vi "3 Phase Generator PMU Testing.vi"() -> ()   [LabVIEW 2022 SP3]
uses:
  <vilib>/Utility/TDMS File Viewer/NI_TDMS File Viewer.lvlib
  <vilib>/measure/NI_MAPro.lvlib
  <vilib>/Waveform/WDTOps.llb/WDT Get Waveform Time Array DBL.vi
panel:
  out "Phase 2":picture caption="Phasors visualization"
  in  "Data type":i32=8
  in  "ROCOF":dbl caption="Offset"
  in  "Data save 2":bool
  in  "Data save":bool
  in  "?":enum32{"Test set-up", "Set up"}(tab)
  out "h2rad":string="rad"
  out "h1rad":string="rad"
  out "h2deg\nH2deg":string="deg"
  out "H1deg":string="deg"
  out "H2V":string="V"
  out "H1V":string="V"
  out "H2pu":string="pu"
  out "H1pu":string="pu"
  out "PMrad":string="rad"
  out "PMdeg":string="deg"
  out "PMFeq":string="Hz"
  out "FreqDev":string="Hz"
  out "second":string="s"
  out "Hz/s":string="Hz/s"
  out "Final freq":string="Hz"
  out "Voltage step (V)":string="V"
  out "Voltage step (pu)":string="pu"
  out "?":string="Hz"
  out "AM (V)":string="V"
  out "AM (pu)":string="pu"
  out "?":string="Hz"
  out "?":string="Hz"
  out "?":string="V"
  out "?":string="pu"
  in  "H2 order":dbl=5.0 format="%#_13g"
  in  "Start":bool
  in  "Final freq.":dbl=55.0 format="%.2f"
  in  "ROCOF rate":dbl=1.0 format="%.2f"
  in  "Select test type":u16(ring) items=["Steady state", "Voltage step", "Phase step", "Frequency step", "Frequency ramp", "Amplitude modulation", "Phase modulation", "Harmonics"]
  in  "Frequency step":dbl caption="Offset" min=-5.0 max=5.0 format="%#.6f"
  in  "Phase step":dbl caption="Offset" min=-360.0 max=360.0 format="%#.6f"
  in  "Phase":dbl caption="Offset" min=-360.0 max=360.0
  in  "Voltage":dbl=1.0 caption="Offset" max=1.25 format="%#_5g"
  in  "Voltage step":dbl caption="Offset" min=-0.25 max=0.25 format="%#.6f"
  in  "Frequency":dbl=50.0 caption="Offset" max=55.0 format="%#_7g"
  in  "Mod Freq":dbl=1.0 caption="Offset" min=0.0 max=2.384 step=0.1 format="%#.6f"
  in  "Mod Amp":dbl=0.1 caption="Offset" max=0.125 format="%#.4f"
  in  "Mod Amp":dbl=0.1 caption="Offset" max=15.0 format="%#.4f"
  in  "Mod Freq":dbl=1.0 caption="Offset" format="%#.6f"
  in  "Nominal voltage":dbl=230.0 caption="Offset" format="%_6f"
  in  "stop":bool
  in  "Phase":dbl caption="Offset"
  in  "H1 Volt":dbl=0.05 format="%#_13g"
  in  "H2 Volt":dbl=0.05 format="%#_13g"
  in  "H1 Phase":dbl format="%#_13g"
  in  "H1 order":dbl=3.0 format="%#_13g"
  in  "H2 Phase":dbl format="%#_13g"
  out "Freq Dev":dbl caption="Offset" max=15.0 format="%#.4f"
  out "ROCOF":dbl
  out "Frequency":dbl=50.0 format="%#.8g"
  out "Voltage":dbl=1.0 format="%#_7g"
  out "Phase":dbl
  out "Phase (rad)":string="rad"
  out "Phase (deg)":string="deg"
  out "Time":dbl
  in  "File Name":string="testfile.tdms" caption="File name"
  in  "start":bool
  out "Phase step (rad)":string="rad"
  out "Phase step (deg)":string="deg"
  in  "Nominal Voltage":dbl=230.0 format="%#_13g"
  out "Transmitted Data":string
  in  "Voltage unit":u16(ring)=1 items=["Nominal voltage", "Per-unit voltage"]
  in  "Phase unit":u16(ring) items=["Degree", "Radian"]
  in  "Sampling info":cluster{"Fs":dbl, "#s":dbl}={"Fs"=10000.0, "#s"=1000.0} {"Fs" format="%.2p"}
  in  "LAN Module IP Address":string
  in  "LAN Port":u16
  in  "Nominal Frequency":dbl=50.0 format="%#_13g"
  out "Phase waveform 2":dbl(graph)
  in  "Initial freq.":dbl=50.0 format="%.2f"
  out "ROCOF waveform 2":dbl(graph)
  out "ROCOF waveform":dynamicdata(graph)
  out "Frequency waveform 2":dbl(graph)
  out "Frequency waveform":dynamicdata(graph)
  out "Votlage waveform":dynamicdata(graph)
  out "Numeric":i32
  out "resulting string 2":string
  out "double precision float":dbl[](array[numeric])
  out "Array 3":dbl[](array[numeric])
  out "Array 2":dbl[](array[numeric])
  out "Array":dbl[](array[numeric])
  out "Phase waveform":waveform(dbl)(graph)
  # "Current phasor values"
  # "UDP Protocol"
  # "Waveform scaling"
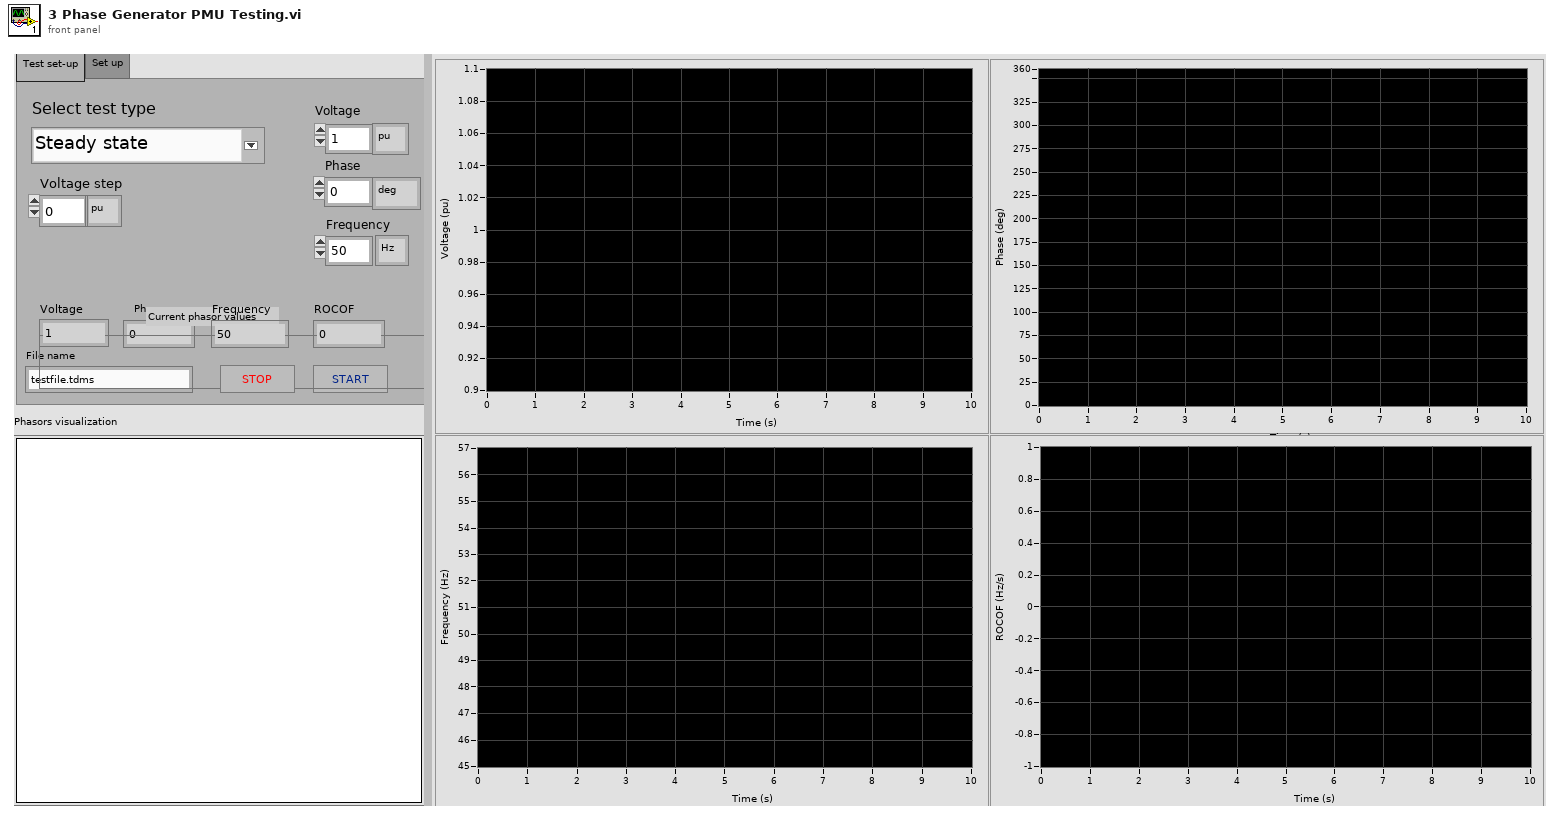
[diagram p1: front panel]
types:
  T1 = enum16{"open", "open or create", "create or replace", "create", "open (read-only)"}
  T2 = cluster{"maximum":dbl, "minimum":dbl, "clip to min":bool, "log?(F)":bool, "grid color":u32, "plot color":u32, "fmt and prec":cluster{"format":enum8{"Decimal", "Scientific", "Engineering", "Binary", "Octal", "Hex"}, "precision":u8}, "visible section":u16}
  T3 = typedef "LVBoundsTypeDef.ctl" = cluster{"Width":u32, "Height":u32}
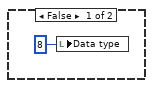
[diagram p2: hidden frame]
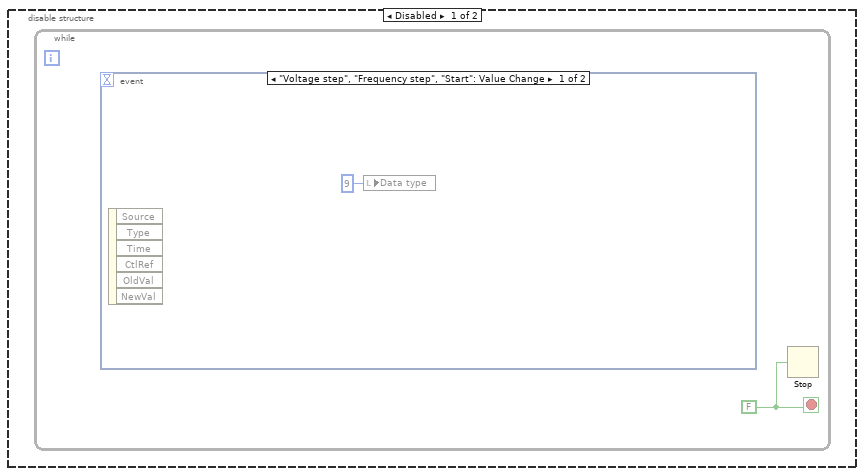
[diagram p3: hidden frame]
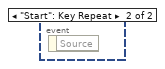
[diagram p4: hidden frame]
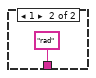
[diagram p5: hidden frame]
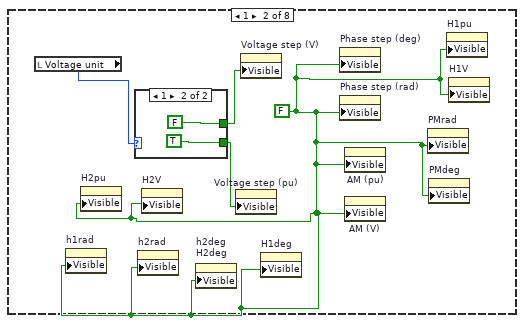
[diagram p6: hidden frame]
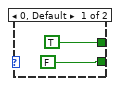
[diagram p7: hidden frame]
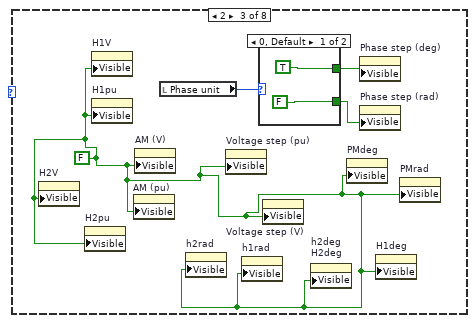
[diagram p8: hidden frame]
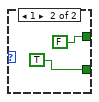
[diagram p9: hidden frame]
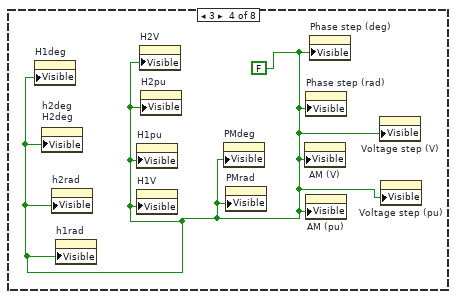
[diagram p10: hidden frame]
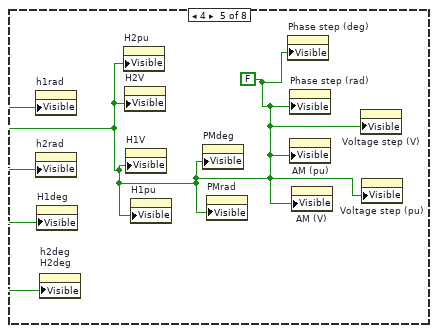
[diagram p11: hidden frame]
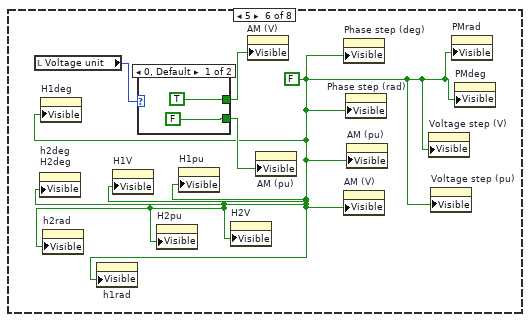
[diagram p12: hidden frame]
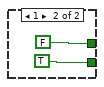
[diagram p13: hidden frame]
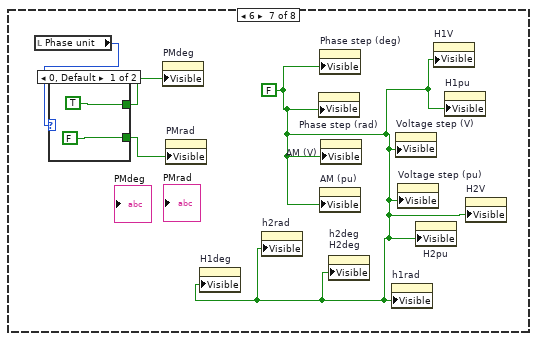
[diagram p14: hidden frame]
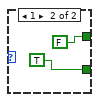
[diagram p15: hidden frame]
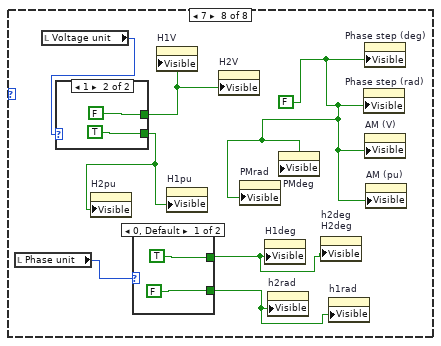
[diagram p16: hidden frame]
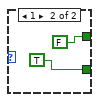
[diagram p17: hidden frame]
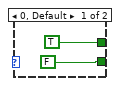
[diagram p18: hidden frame]
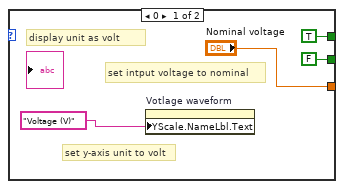
[diagram p19: hidden frame]
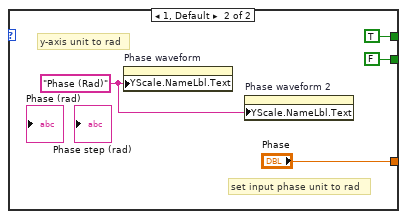
[diagram p20: hidden frame]
diagram:
  n1 = call <vilib>:"Application Directory.vi"() -> ("Application Directory"=w5:path)
  n2 = Concatenate Strings("measurements\\", "File Name") -> (w3:string)
  n3 = Build Path(base path=w5, name or relative path=w3) -> (appended path=w4:path)
  n4 = flat-sequence {
    frame #0 {
      w23 = FALSE
      n5 = local read "Data type"() -> (w29:i32)
      n6 = local read "start"() -> (w22:bool)
      n7 = Equal?(x=w29, y=8) -> (x = y?=w28:bool)
      n8 = Equal?(x=w22, y=TRUE) -> (x = y?=w27:bool)
      n9 = And(x=w27, y=w28) -> (x .and. y?=w26:bool)
      n10 = case shown="True" w26 {
        frame False {
          n11 = local write "Data type"(8 ("Data type")) -> ()
        }
        frame True {
          n12 = local write "Data type"(9 ("Data type")) -> ()
        }
      }
      n13 = property on="Start" class="Bool (strict)"("Value"=w23) -> ()  [unwired: 2 in, 2 out]
      n14 = property on="start" class="Bool (strict)"("Value"=w23) -> ()  [unwired: 2 in, 2 out]
    }
  }
  n15 = TDMS Open(10:T1."create or replace" ("operation (0:open)"), 11:w4) -> (0:w14:errorcluster, 3:w15:refnum<k34>)  [unwired: 5 in]
  n16 = TDMS Set Properties(5:"Data file for PMU testing", 7:"title", 8:w14, 11:w15) -> (0:w12:errorcluster, 3:w13:refnum<k34>)  [unwired: 2 in, 2 out]
  n17 = Get Date/Time In Seconds() -> (seconds since 1Jan1904=w16:timestamp)
  n18 = TDMS Set Properties(5:w16, 7:"datetime", 8:w12, 11:w13) -> (0:w7:errorcluster, 3:w6:refnum<k34>)  [unwired: 2 in, 2 out]
  n19 = while {
    tunnel: [w37] -> w18
    tunnel: [w36] -> w17
    tunnel: w7 -> [w34]
    tunnel: w6 -> [w35]
    i -> [w69]
    stop <- "stop" stop-if-true
    w44 = "3 Phase Generator" ("group name in (Untitled)")
    # "amplitude modulation\nmod freq unit"
    # "phase \nmodulation\namplitude \nunit"
    # "stop button"
    # "box for config layout"
    n20 = flat-sequence {
      tunnel: ["start"] -> w40
      tunnel: ["start"] -> _
      tunnel: [w87] -> w43
      tunnel: [w82] -> w42
      tunnel: [w85] -> w41
      tunnel: w40 -> [w87]
      tunnel: [w166] -> w74
      tunnel: w43 -> [w166]
      tunnel: w42 -> [w160]
      tunnel: w41 -> [w178]
      tunnel: w39 -> [w174]
      tunnel: w38 -> [w173]
      tunnel: [w172] -> w37
      tunnel: [w171] -> w36
      tunnel: w74 -> [w738]
      frame #0 {
        # "input freq unit"
        # "start button"
      }
      frame #1 {
        # "voltage step"
        # "amplitude modulation unit"
        # "set default angle unit ot rad\nif input deg, convert to rad"
        # "enable nominal voltage"
        # "enable unit volt"
        # "enable unit per-unit"
        # "enable per-unit voltage"
        # "per-unit voltage or nominal voltage"
        n21 = local read "Select test type"() -> (w80:u16)
        n22 = case shown="0" "Phase unit" {
          tunnel: [w147 "Phase"] -> w82
          tunnel: [FALSE TRUE] -> w78
          tunnel: [TRUE FALSE] -> w79
          frame 0 {
            # "convert deg to rad"
            # "y-axis in deg"
            # "set input phase unit to deg"
            n23 = property on="Phase waveform" class="WFChart (strict)"("YScale.NameLbl.Text"="Phase (deg)" ("Y Scale.Name Label.Text")) -> ()  [unwired: 2 in, 2 out]
            n24 = Multiply(x="Phase", y=3.141592653589793) -> (x*y=w150:dbl)
            n25 = Divide(x=w150, y=180.0) -> (x/y=w147:dbl)
          }
          frame 1, Default {
            w154 = "Phase (Rad)" ("Y Scale.Name Label.Text")
            # "y-axis unit to rad"
            # "set input phase unit to rad"
            n26 = property on="Phase waveform" class="WFChart (strict)"("YScale.NameLbl.Text"=w154) -> ()  [unwired: 2 in, 2 out]
            n27 = property on="Phase waveform 2" class="WFChart (strict)"("YScale.NameLbl.Text"=w154) -> ()  [unwired: 2 in, 2 out]
          }
        }
        n28 = case shown="0, Default" w80 {
          frame 0, Default {
            w88 = FALSE
            n29 = property on="H2V" class="Str"("Visible"=w88) -> ()  [unwired: 2 in, 2 out]
            n30 = property on="H2pu" class="Str"("Visible"=w88) -> ()  [unwired: 2 in, 2 out]
            n31 = property on="h1rad" class="Str"("Visible"=w88) -> ()  [unwired: 2 in, 2 out]
            n32 = property on="H1deg" class="Str"("Visible"=w88) -> ()  [unwired: 2 in, 2 out]
            n33 = property on="H1V" class="Str"("Visible"=w88) -> ()  [unwired: 2 in, 2 out]
            n34 = property on="H1pu" class="Str"("Visible"=w88) -> ()  [unwired: 2 in, 2 out]
            n35 = property on="h2rad" class="Str"("Visible"=w88) -> ()  [unwired: 2 in, 2 out]
            n36 = property on="h2deg\nH2deg" class="Str"("Visible"=w88) -> ()  [unwired: 2 in, 2 out]
            n37 = property on="PMdeg" class="Str"("Visible"=w88) -> ()  [unwired: 2 in, 2 out]
            n38 = property on="PMrad" class="Str"("Visible"=w88) -> ()  [unwired: 2 in, 2 out]
            n39 = property on="Voltage step (pu)" class="Str"("Visible"=w88) -> ()  [unwired: 2 in, 2 out]
            n40 = property on="AM (pu)" class="Str"("Visible"=w88) -> ()  [unwired: 2 in, 2 out]
            n41 = property on="AM (V)" class="Str"("Visible"=w88) -> ()  [unwired: 2 in, 2 out]
            n42 = property on="Phase step (deg)" class="Str"("Visible"=w88) -> ()  [unwired: 2 in, 2 out]
            n43 = property on="Phase step (rad)" class="Str"("Visible"=w88) -> ()  [unwired: 2 in, 2 out]
            n44 = property on="Voltage step (V)" class="Str"("Visible"=w88) -> ()  [unwired: 2 in, 2 out]
          }
          frame 1 {
            w89 = FALSE
            n45 = local read "Voltage unit"() -> (w92:u16)
            n46 = property on="h1rad" class="Str"("Visible"=w89) -> ()  [unwired: 2 in, 2 out]
            n47 = property on="H2pu" class="Str"("Visible"=w89) -> ()  [unwired: 2 in, 2 out]
            n48 = case shown="1" w92 {
              tunnel: [TRUE FALSE] -> w90
              tunnel: [FALSE TRUE] -> w91
              frame 0, Default {
              }
              frame 1 {
              }
            }
            n49 = property on="h2rad" class="Str"("Visible"=w89) -> ()  [unwired: 2 in, 2 out]
            n50 = property on="H2V" class="Str"("Visible"=w89) -> ()  [unwired: 2 in, 2 out]
            n51 = property on="h2deg\nH2deg" class="Str"("Visible"=w89) -> ()  [unwired: 2 in, 2 out]
            n52 = property on="Voltage step (pu)" class="Str"("Visible"=w91) -> ()  [unwired: 2 in, 2 out]
            n53 = property on="Voltage step (V)" class="Str"("Visible"=w90) -> ()  [unwired: 2 in, 2 out]
            n54 = property on="H1deg" class="Str"("Visible"=w89) -> ()  [unwired: 2 in, 2 out]
            n55 = property on="Phase step (deg)" class="Str"("Visible"=w89) -> ()  [unwired: 2 in, 2 out]
            n56 = property on="Phase step (rad)" class="Str"("Visible"=w89) -> ()  [unwired: 2 in, 2 out]
            n57 = property on="AM (pu)" class="Str"("Visible"=w89) -> ()  [unwired: 2 in, 2 out]
            n58 = property on="AM (V)" class="Str"("Visible"=w89) -> ()  [unwired: 2 in, 2 out]
            n59 = property on="PMrad" class="Str"("Visible"=w89) -> ()  [unwired: 2 in, 2 out]
            n60 = property on="PMdeg" class="Str"("Visible"=w89) -> ()  [unwired: 2 in, 2 out]
            n61 = property on="H1pu" class="Str"("Visible"=w89) -> ()  [unwired: 2 in, 2 out]
            n62 = property on="H1V" class="Str"("Visible"=w89) -> ()  [unwired: 2 in, 2 out]
          }
          frame 2 {
            w97 = FALSE
            n63 = property on="H2V" class="Str"("Visible"=w97) -> ()  [unwired: 2 in, 2 out]
            n64 = property on="H2pu" class="Str"("Visible"=w97) -> ()  [unwired: 2 in, 2 out]
            n65 = property on="H1V" class="Str"("Visible"=w97) -> ()  [unwired: 2 in, 2 out]
            n66 = property on="H1pu" class="Str"("Visible"=w97) -> ()  [unwired: 2 in, 2 out]
            n67 = property on="AM (pu)" class="Str"("Visible"=w97) -> ()  [unwired: 2 in, 2 out]
            n68 = property on="AM (V)" class="Str"("Visible"=w97) -> ()  [unwired: 2 in, 2 out]
            n69 = local read "Phase unit"() -> (w98:u16)
            n70 = property on="h2rad" class="Str"("Visible"=w97) -> ()  [unwired: 2 in, 2 out]
            n71 = property on="Voltage step (pu)" class="Str"("Visible"=w97) -> ()  [unwired: 2 in, 2 out]
            n72 = property on="h1rad" class="Str"("Visible"=w97) -> ()  [unwired: 2 in, 2 out]
            n73 = case shown="0, Default" w98 {
              tunnel: [TRUE FALSE] -> w100
              tunnel: [FALSE TRUE] -> w99
              frame 0, Default {
              }
              frame 1 {
              }
            }
            n74 = property on="Voltage step (V)" class="Str"("Visible"=w97) -> ()  [unwired: 2 in, 2 out]
            n75 = property on="h2deg\nH2deg" class="Str"("Visible"=w97) -> ()  [unwired: 2 in, 2 out]
            n76 = property on="PMdeg" class="Str"("Visible"=w97) -> ()  [unwired: 2 in, 2 out]
            n77 = property on="Phase step (deg)" class="Str"("Visible"=w100) -> ()  [unwired: 2 in, 2 out]
            n78 = property on="Phase step (rad)" class="Str"("Visible"=w99) -> ()  [unwired: 2 in, 2 out]
            n79 = property on="H1deg" class="Str"("Visible"=w97) -> ()  [unwired: 2 in, 2 out]
            n80 = property on="PMrad" class="Str"("Visible"=w97) -> ()  [unwired: 2 in, 2 out]
          }
          frame 3 {
            w105 = FALSE
            n81 = property on="H1deg" class="Str"("Visible"=w105) -> ()  [unwired: 2 in, 2 out]
            n82 = property on="h2deg\nH2deg" class="Str"("Visible"=w105) -> ()  [unwired: 2 in, 2 out]
            n83 = property on="h2rad" class="Str"("Visible"=w105) -> ()  [unwired: 2 in, 2 out]
            n84 = property on="h1rad" class="Str"("Visible"=w105) -> ()  [unwired: 2 in, 2 out]
            n85 = property on="H1pu" class="Str"("Visible"=w105) -> ()  [unwired: 2 in, 2 out]
            n86 = property on="H1V" class="Str"("Visible"=w105) -> ()  [unwired: 2 in, 2 out]
            n87 = property on="H2V" class="Str"("Visible"=w105) -> ()  [unwired: 2 in, 2 out]
            n88 = property on="H2pu" class="Str"("Visible"=w105) -> ()  [unwired: 2 in, 2 out]
            n89 = property on="PMdeg" class="Str"("Visible"=w105) -> ()  [unwired: 2 in, 2 out]
            n90 = property on="PMrad" class="Str"("Visible"=w105) -> ()  [unwired: 2 in, 2 out]
            n91 = property on="AM (V)" class="Str"("Visible"=w105) -> ()  [unwired: 2 in, 2 out]
            n92 = property on="Phase step (rad)" class="Str"("Visible"=w105) -> ()  [unwired: 2 in, 2 out]
            n93 = property on="AM (pu)" class="Str"("Visible"=w105) -> ()  [unwired: 2 in, 2 out]
            n94 = property on="Phase step (deg)" class="Str"("Visible"=w105) -> ()  [unwired: 2 in, 2 out]
            n95 = property on="Voltage step (V)" class="Str"("Visible"=w105) -> ()  [unwired: 2 in, 2 out]
            n96 = property on="Voltage step (pu)" class="Str"("Visible"=w105) -> ()  [unwired: 2 in, 2 out]
          }
          frame 4 {
            w106 = FALSE
            n97 = property on="h1rad" class="Str"("Visible"=w106) -> ()  [unwired: 2 in, 2 out]
            n98 = property on="h2rad" class="Str"("Visible"=w106) -> ()  [unwired: 2 in, 2 out]
            n99 = property on="H1deg" class="Str"("Visible"=w106) -> ()  [unwired: 2 in, 2 out]
            n100 = property on="h2deg\nH2deg" class="Str"("Visible"=w106) -> ()  [unwired: 2 in, 2 out]
            n101 = property on="H2pu" class="Str"("Visible"=w106) -> ()  [unwired: 2 in, 2 out]
            n102 = property on="H2V" class="Str"("Visible"=w106) -> ()  [unwired: 2 in, 2 out]
            n103 = property on="H1V" class="Str"("Visible"=w106) -> ()  [unwired: 2 in, 2 out]
            n104 = property on="H1pu" class="Str"("Visible"=w106) -> ()  [unwired: 2 in, 2 out]
            n105 = property on="PMdeg" class="Str"("Visible"=w106) -> ()  [unwired: 2 in, 2 out]
            n106 = property on="PMrad" class="Str"("Visible"=w106) -> ()  [unwired: 2 in, 2 out]
            n107 = property on="Phase step (deg)" class="Str"("Visible"=w106) -> ()  [unwired: 2 in, 2 out]
            n108 = property on="Phase step (rad)" class="Str"("Visible"=w106) -> ()  [unwired: 2 in, 2 out]
            n109 = property on="AM (pu)" class="Str"("Visible"=w106) -> ()  [unwired: 2 in, 2 out]
            n110 = property on="AM (V)" class="Str"("Visible"=w106) -> ()  [unwired: 2 in, 2 out]
            n111 = property on="Voltage step (V)" class="Str"("Visible"=w106) -> ()  [unwired: 2 in, 2 out]
            n112 = property on="Voltage step (pu)" class="Str"("Visible"=w106) -> ()  [unwired: 2 in, 2 out]
          }
          frame 5 {
            w107 = FALSE
            n113 = local read "Voltage unit"() -> (w110:u16)
            n114 = property on="h2deg\nH2deg" class="Str"("Visible"=w107) -> ()  [unwired: 2 in, 2 out]
            n115 = property on="H1deg" class="Str"("Visible"=w107) -> ()  [unwired: 2 in, 2 out]
            n116 = property on="h2rad" class="Str"("Visible"=w107) -> ()  [unwired: 2 in, 2 out]
            n117 = property on="h1rad" class="Str"("Visible"=w107) -> ()  [unwired: 2 in, 2 out]
            n118 = property on="H1V" class="Str"("Visible"=w107) -> ()  [unwired: 2 in, 2 out]
            n119 = case shown="0, Default" w110 {
              tunnel: [TRUE FALSE] -> w109
              tunnel: [FALSE TRUE] -> w108
              frame 0, Default {
              }
              frame 1 {
              }
            }
            n120 = property on="H2pu" class="Str"("Visible"=w107) -> ()  [unwired: 2 in, 2 out]
            n121 = property on="H1pu" class="Str"("Visible"=w107) -> ()  [unwired: 2 in, 2 out]
            n122 = property on="H2V" class="Str"("Visible"=w107) -> ()  [unwired: 2 in, 2 out]
            n123 = property on="AM (V)" class="Str"("Visible"=w109) -> ()  [unwired: 2 in, 2 out]
            n124 = property on="AM (pu)" class="Str"("Visible"=w108) -> ()  [unwired: 2 in, 2 out]
            n125 = property on="Phase step (deg)" class="Str"("Visible"=w107) -> ()  [unwired: 2 in, 2 out]
            n126 = property on="AM (V)" class="Str"("Visible"=w107) -> ()  [unwired: 2 in, 2 out]
            n127 = property on="Phase step (rad)" class="Str"("Visible"=w107) -> ()  [unwired: 2 in, 2 out]
            n128 = property on="AM (pu)" class="Str"("Visible"=w107) -> ()  [unwired: 2 in, 2 out]
            n129 = property on="Voltage step (V)" class="Str"("Visible"=w107) -> ()  [unwired: 2 in, 2 out]
            n130 = property on="Voltage step (pu)" class="Str"("Visible"=w107) -> ()  [unwired: 2 in, 2 out]
            n131 = property on="PMrad" class="Str"("Visible"=w107) -> ()  [unwired: 2 in, 2 out]
            n132 = property on="PMdeg" class="Str"("Visible"=w107) -> ()  [unwired: 2 in, 2 out]
          }
          frame 6 {
            w115 = FALSE
            n133 = local read "Phase unit"() -> (w118:u16)
            n134 = case shown="0, Default" w118 {
              tunnel: [TRUE FALSE] -> w117
              tunnel: [FALSE TRUE] -> w116
              frame 0, Default {
              }
              frame 1 {
              }
            }
            n135 = property on="PMdeg" class="Str"("Visible"=w117) -> ()  [unwired: 2 in, 2 out]
            n136 = property on="PMrad" class="Str"("Visible"=w116) -> ()  [unwired: 2 in, 2 out]
            n137 = property on="H1deg" class="Str"("Visible"=w115) -> ()  [unwired: 2 in, 2 out]
            n138 = property on="h2rad" class="Str"("Visible"=w115) -> ()  [unwired: 2 in, 2 out]
            n139 = property on="Phase step (rad)" class="Str"("Visible"=w115) -> ()  [unwired: 2 in, 2 out]
            n140 = property on="Phase step (deg)" class="Str"("Visible"=w115) -> ()  [unwired: 2 in, 2 out]
            n141 = property on="AM (pu)" class="Str"("Visible"=w115) -> ()  [unwired: 2 in, 2 out]
            n142 = property on="AM (V)" class="Str"("Visible"=w115) -> ()  [unwired: 2 in, 2 out]
            n143 = property on="h2deg\nH2deg" class="Str"("Visible"=w115) -> ()  [unwired: 2 in, 2 out]
            n144 = property on="h1rad" class="Str"("Visible"=w115) -> ()  [unwired: 2 in, 2 out]
            n145 = property on="Voltage step (V)" class="Str"("Visible"=w115) -> ()  [unwired: 2 in, 2 out]
            n146 = property on="Voltage step (pu)" class="Str"("Visible"=w115) -> ()  [unwired: 2 in, 2 out]
            n147 = property on="H2pu" class="Str"("Visible"=w115) -> ()  [unwired: 2 in, 2 out]
            n148 = property on="H1V" class="Str"("Visible"=w115) -> ()  [unwired: 2 in, 2 out]
            n149 = property on="H1pu" class="Str"("Visible"=w115) -> ()  [unwired: 2 in, 2 out]
            n150 = property on="H2V" class="Str"("Visible"=w115) -> ()  [unwired: 2 in, 2 out]
          }
          frame 7 {
            w129 = FALSE
            n151 = local read "Phase unit"() -> (w123:u16)
            n152 = local read "Voltage unit"() -> (w128:u16)
            n153 = case shown="1" w128 {
              tunnel: [TRUE FALSE] -> w127
              tunnel: [FALSE TRUE] -> w126
              frame 0, Default {
              }
              frame 1 {
              }
            }
            n154 = property on="H2pu" class="Str"("Visible"=w126) -> ()  [unwired: 2 in, 2 out]
            n155 = case shown="0, Default" w123 {
              tunnel: [TRUE FALSE] -> w125
              tunnel: [FALSE TRUE] -> w124
              frame 0, Default {
              }
              frame 1 {
              }
            }
            n156 = property on="H1V" class="Str"("Visible"=w127) -> ()  [unwired: 2 in, 2 out]
            n157 = property on="H1pu" class="Str"("Visible"=w126) -> ()  [unwired: 2 in, 2 out]
            n158 = property on="H2V" class="Str"("Visible"=w127) -> ()  [unwired: 2 in, 2 out]
            n159 = property on="PMrad" class="Str"("Visible"=w129) -> ()  [unwired: 2 in, 2 out]
            n160 = property on="H1deg" class="Str"("Visible"=w125) -> ()  [unwired: 2 in, 2 out]
            n161 = property on="h2rad" class="Str"("Visible"=w124) -> ()  [unwired: 2 in, 2 out]
            n162 = property on="PMdeg" class="Str"("Visible"=w129) -> ()  [unwired: 2 in, 2 out]
            n163 = property on="h2deg\nH2deg" class="Str"("Visible"=w125) -> ()  [unwired: 2 in, 2 out]
            n164 = property on="h1rad" class="Str"("Visible"=w124) -> ()  [unwired: 2 in, 2 out]
            n165 = property on="Phase step (rad)" class="Str"("Visible"=w129) -> ()  [unwired: 2 in, 2 out]
            n166 = property on="Phase step (deg)" class="Str"("Visible"=w129) -> ()  [unwired: 2 in, 2 out]
            n167 = property on="AM (V)" class="Str"("Visible"=w129) -> ()  [unwired: 2 in, 2 out]
            n168 = property on="AM (pu)" class="Str"("Visible"=w129) -> ()  [unwired: 2 in, 2 out]
          }
        }
        n169 = case shown="1, Default" "Voltage unit" {
          tunnel: ["Nominal voltage" "Voltage"] -> w85
          tunnel: [TRUE FALSE] -> w83
          tunnel: [FALSE TRUE] -> w84
          frame 0 {
            # "set intput voltage to nominal"
            # "display unit as volt"
            # "set y-axis unit to volt"
            n170 = property on="Votlage waveform" class="WFChart (strict)"("YScale.NameLbl.Text"="Voltage (V)" ("Y Scale.Name Label.Text")) -> ()  [unwired: 2 in, 2 out]
          }
          frame 1, Default {
            # "set voltage unit to pu"
            # "set y-axis to show in per-unit scale"
            n171 = property on="Votlage waveform" class="WFChart (strict)"("YScale.NameLbl.Text"="Voltage (pu)" ("Y Scale.Name Label.Text")) -> ()  [unwired: 2 in, 2 out]
          }
        }
        n172 = property on="AM (pu)" class="Str" props=["Visible"]() -> ()  [unwired: 2 in, 3 out]
        n173 = property on="AM (pu)" class="Str" props=["Visible"]() -> ()  [unwired: 2 in, 3 out]
        n174 = property on="Phase (deg)" class="Str"("Visible"=w79) -> ()  [unwired: 2 in, 2 out]
        n175 = property on="Phase (rad)" class="Str"("Visible"=w78) -> ()  [unwired: 2 in, 2 out]
        n176 = property class="Str"("Visible"=w84) -> ()  [unwired: 2 in, 2 out]
        n177 = property on="Nominal voltage" class="DigNum (strict)"("Visible"=w83) -> ()  [unwired: 2 in, 2 out]
        n178 = property class="Str"("Visible"=w83) -> ()  [unwired: 2 in, 2 out]
        n179 = property on="Voltage" class="DigNum (strict)"("Visible"=w84) -> ()  [unwired: 2 in, 2 out]
        n180 = property on="Phase (rad)" class="DigNum (strict)"("Visible"=w78) -> ()  [unwired: 2 in, 2 out]
        n181 = property on="Phase (deg)" class="DigNum (strict)"("Visible"=w79) -> ()  [unwired: 2 in, 2 out]
        n182 = invoke on="double precision float" class="Arr (strict)" method="Reinit To Default"() -> ()  [unwired: 3 in, 3 out]
      }
      frame #2 {
        # "phase in"
        # "voltage in"
        # "start generating"
        n183 = invoke on="Array 3" class="Arr (strict)" method="Reinit To Default"() -> ()  [unwired: 3 in, 3 out]
        n184 = invoke on="Array 2" class="Arr (strict)" method="Reinit To Default"() -> ()  [unwired: 3 in, 3 out]
        n185 = invoke on="Array" class="Arr (strict)" method="Reinit To Default"() -> ()  [unwired: 3 in, 3 out]
        n186 = case shown="True" w166 {
          selector: w166 -> [_ w255]
          tunnel: "Select test type" -> [w224 w263]
          tunnel: [w220 w260] -> w163
          tunnel: [w223 w251] -> w176
          tunnel: [w218 w248] -> _
          tunnel: [w217 w252] -> w158
          tunnel: [w215 w249] -> w164
          tunnel: [w219 w250] -> w165
          tunnel: [w216 w259] -> w159
          tunnel: [w221 w258] -> _
          tunnel: [w222 w257] -> w162
          tunnel: [w209 w256] -> w161
          tunnel: w160 -> [_ w254]
          tunnel: w178 -> [_ w253]
          tunnel: [w214 w247] -> w177
          tunnel: [w213 w246] -> w175
          tunnel: [w212 w245] -> w170
          tunnel: [w212 w244] -> w169
          tunnel: [w212 w243] -> w168
          tunnel: [w212 w242] -> w167
          frame False {
            w210 = dbl[] [] ("History Data")
            w212 = dbl[] []
            w211 = waveform(dbl)[] [] ("History Data")
            n187 = property on="Frequency waveform 2" class="WFChart (strict)"("History Data"=w210) -> ()  [unwired: 2 in, 2 out]
            n188 = property on="ROCOF waveform 2" class="WFChart (strict)"("History Data"=w210) -> ()  [unwired: 2 in, 2 out]
            n189 = property on="Phase waveform 2" class="WFChart (strict)"("History Data"=w210) -> ()  [unwired: 2 in, 2 out]
            n190 = property on="Frequency waveform" class="WFChart (strict)"("History Data"=w211) -> ()  [unwired: 2 in, 2 out]
            n191 = property on="Phase waveform" class="WFChart (strict)"("History Data"=w211) -> ()  [unwired: 2 in, 2 out]
            n192 = property on="Votlage waveform" class="WFChart (strict)"("History Data"=w211) -> ()  [unwired: 2 in, 2 out]
            n193 = property on="ROCOF waveform" class="WFChart (strict)"("History Data"=w211) -> ()  [unwired: 2 in, 2 out]
            n194 = case shown="0, Default" w224 {
              tunnel: [w226 w228 w229 w231 w234 w236 w238 w239] -> _
              tunnel: [w226 w228 w229 w231 w234 w236 w238 w240] -> w223
              tunnel: [w225 w227 w230 w232 w233 w236 w237 w239] -> w222
              tunnel: [w225 w227 w230 w232 w233 w235 w238 w239] -> w209
              tunnel: [w225 w227 w230 w232 w233 w235 w237 w239] -> w221
              tunnel: [w225 w227 w229 w232 w233 w235 w237 w239] -> w220
              tunnel: [w225 w227 w230 w231 w233 w235 w237 w239] -> w219
              tunnel: [w225 w227 w230 w232 w233 w235 w237 w239] -> w218
              tunnel: [w225 w227 w230 w232 w233 w235 w237 w240] -> w215
              tunnel: [w225 w228 w230 w232 w233 w235 w237 w239] -> w217
              tunnel: [w225 w227 w230 w232 w234 w235 w237 w239] -> w216
              tunnel: [w225 w227 w229 w232 w233 w235 w237 w239] -> w214
              tunnel: [w225 w227 w229 w231 w233 w235 w237 w239] -> w213
              frame 0, Default {
                w226 = TRUE
                w225 = FALSE
              }
              frame 1 {
                w228 = TRUE
                w227 = FALSE
              }
              frame 2 {
                w229 = TRUE
                w230 = FALSE
              }
              frame 3 {
                w231 = TRUE
                w232 = FALSE
              }
              frame 4 {
                w234 = TRUE
                w233 = FALSE
              }
              frame 5 {
                w236 = TRUE
                w235 = FALSE
              }
              frame 6 {
                w238 = TRUE
                w237 = FALSE
              }
              frame 7 {
                w239 = FALSE
                w240 = TRUE
              }
            }
          }
          frame True {
            # "phase mod freq dev unit"
            # "phase mod freq unit"
            n195 = case shown="0, Default" w263 {
              tunnel: w253 -> [w296 w319 w380 w447 w550 w636 w707 w735]
              tunnel: w254 -> [w274 w304 w378 w456 w563 w651 w682 _]
              tunnel: "Frequency" -> [w275 w306 w362 w461 w545 w648 w683 w737]
              tunnel: "ROCOF" -> [w290 w323 w358 w440 _ w647 w681 _]
              tunnel: [w279 w333 w369 w446 w579 w659 w713 w734] -> _
              tunnel: [w289 w311 w369 w449 w546 w634 w680 w734] -> w260
              tunnel: [w279 w333 w369 w446 w579 w659 w713 w736] -> w251
              tunnel: [w289 w311 w369 w449 w546 w659 w713 w736] -> w248
              tunnel: [w279 w333 w369 w446 w579 w659 w713 w734] -> _
              tunnel: [w289 w311 w392 w449 w546 w634 w680 w736] -> w249
              tunnel: [w289 w311 w392 w446 w546 w634 w680 w734] -> w250
              tunnel: [w289 w311 w392 w449 w579 w634 w680 w734] -> w259
              tunnel: [w289 w311 w392 w449 w546 w634 w680 w734] -> w258
              tunnel: [w289 w311 w392 w449 w546 w659 w680 w734] -> w257
              tunnel: [w289 w311 w392 w449 w546 w634 w713 w734] -> w256
              tunnel: w255 -> [_ _ _ _ _ _ _ _]
              tunnel: [w289 w333 w392 w449 w546 w634 w680 w734] -> w252
              tunnel: [w289 w311 w369 w449 w546 w634 w680 w734] -> w247
              tunnel: [w279 w311 w369 w446 w546 w634 w680 w734] -> w246
              tunnel: [w285 w307 w365 w435 w539 w630 w676 w733] -> w245
              tunnel: [w286 w309 w363 w444 w544 w629 w673 w733] -> w244
              tunnel: [w266 w308 w364 w436 w542 w632 w674 w733] -> w243
              tunnel: [w277 w310 w366 w443 w528 w631 w675 w733] -> w242
              tunnel: "Nominal Frequency" -> [w267 w305 w339 _ _ _ _ _]
              frame 0, Default {
                w279 = TRUE
                w289 = FALSE
                # "nominal freq"
                # "delta rocof = differenciate delta freq"
                # "rocof func: f(t)=rocof"
                # "input freq: f(t)=f_in"
                # "voltage in func: f(t)=v_in"
                # "Steady state"
                n196 = local read "Sampling info"() -> (w264:cluster{"Fs":dbl, "#s":dbl})
                n197 = local read "Phase unit"() -> (w273:u16)
                n198 = call "phasePlotWrap.vi"("Sampling info"=w264, "Phase unit"=w273, "Phase"=w274, "Nominal Frequency"=w267, "Frequency"=w275) -> ("yScaleMin"=w270:dbl, "yScaleMax"=w271:dbl, "Phase waveform"=w272:waveform(dbl))  [unwired: 4 in]
                "Phase waveform" <- w272
                n199 = call "Convert to Dynamic Data"("Array"=w272) -> ("Dynamic Data Type"=w276:dynamicdata)  [unwired: 3 in]
                n200 = call "Convert from Dynamic Data13"("Dynamic Data Type"=w276) -> ("Array"=w285:dbl[])  [unwired: 3 in]
                n201 = call <vilib>:"Formula Waveform.vi"("sampling info"=w264, "formula"="a", "amplitude"=w275) -> ("signal out"=w266:waveform(dbl))  [unwired: 7 in, 1 out]
                n202 = call <vilib>:"Formula Waveform.vi"("sampling info"=w264, "formula"="a", "frequency"=w267) -> ("signal out"=w268:waveform(dbl))  [unwired: 7 in, 1 out]
                n203 = Subtract(1:w268, 2:w266) -> (0:w265:waveform(dbl))  [unwired: 1 in, 1 out]
                n204 = property on="Phase waveform" class="WFChart (strict)"("YScale.Maximum"=w271) -> ()  [unwired: 2 in, 2 out]
                n205 = property on="Phase waveform" class="WFChart (strict)"("YScale.Minimum"=w270) -> ()  [unwired: 2 in, 2 out]
                n206 = call "Sample Compression8"("Signals"=w266) -> ("Maximum"=w291:dynamicdata)  [unwired: 8 in, 2 out]
                "Frequency waveform" <- w291
                n207 = call "Derivative (dX/dt)"("Signals"=w265) -> ("Result"=w278:dynamicdata)  [unwired: 5 in, 1 out]
                n208 = call "Convert from Dynamic Data3"("Dynamic Data Type"=w278) -> ("Array"=w277:dbl[])  [unwired: 3 in]
                n209 = call <vilib>:"Formula Waveform.vi"("sampling info"=w264, "formula"="a", "amplitude"=w290) -> ("signal out"=w288:waveform(dbl))  [unwired: 7 in, 1 out]
                n210 = local write "Phase"(w272) -> ()
                n211 = call-poly <vilib>:"Get Waveform Time Array.vi"("waveform in"=w288) -> ("X array"=w293:timestamp[])  [unwired: 9 in, 1 out]
                n212 = local write "Frequency"(w291) -> ()
                n213 = call <vilib>:"Formula Waveform.vi"("sampling info"=w264, "formula"="a", "amplitude"=w296) -> ("signal out"=w286:waveform(dbl))  [unwired: 7 in, 1 out]
                n214 = To Double Precision Float(number=w293) -> (double precision float=→"double precision float":dbl[])
                n215 = call "Sample Compression6"("Signals"=w286) -> ("Maximum"=w292:dynamicdata)  [unwired: 8 in, 2 out]
                "Votlage waveform" <- w292
                n216 = call "Sample Compression50"("Signals"=w278) -> ("Maximum"=w280:dynamicdata)  [unwired: 8 in, 2 out]
                "ROCOF" <- w280
                n217 = call "Convert from Dynamic Data10"("Dynamic Data Type"=w280) -> ("Scalar"=w284:dbl)  [unwired: 3 in]
                n218 = local write "Voltage"(w292) -> ()
                n219 = In Range and Coerce(upper limit=5.0, x=w284, lower limit=-5.0) -> (coerced(x)=w281:dbl)  [unwired: 1 out]
                n220 = local write "ROCOF waveform 2"(w281) -> ()
                n221 = call "Elapsed Time3"() -> ("Time has Elapsed"=w287:bool)  [unwired: 12 in, 7 out]
                n222 = Stop(stop? (T)=w287) -> ()
              }
              frame 1 {
                w311 = FALSE
                w333 = TRUE ("Visible")
                # "because the compression remove half of the sample so the last 0.1s will turn to 0.05s, delay 1s will be 0.95s instead"
                # "input freq"
                # "initial phase"
                # "percentage of the base voltage"
                # "base voltage"
                # "voltage step"
                n223 = local read "Sampling info"() -> (w302:cluster{"Fs":dbl, "#s":dbl})
                n224 = call <vilib>:"Formula Waveform.vi"("sampling info"=w302, "formula"="a", "amplitude"=w306) -> ("signal out"=w308:waveform(dbl))  [unwired: 7 in, 1 out]
                n225 = call <vilib>:"Formula Waveform.vi"("sampling info"=w302, "formula"="a", "amplitude"=w304) -> ("signal out"=w307:waveform(dbl))  [unwired: 7 in, 1 out]
                n226 = call "Sample Compression9"("Signals"=w308) -> ("Maximum"=w316:dynamicdata)  [unwired: 8 in, 2 out]
                n227 = local write "Array 2"(w307) -> ()
                n228 = call <vilib>:"Formula Waveform.vi"("sampling info"=w302, "formula"="a", "amplitude"=w319) -> ("signal out"=w313:waveform(dbl))  [unwired: 7 in, 1 out]
                n229 = call <vilib>:"Formula Waveform.vi"("sampling info"=w302, "formula"="a", "amplitude"=w323) -> ("signal out"=w310:waveform(dbl))  [unwired: 7 in, 1 out]
                n230 = call <vilib>:"Formula Waveform.vi"("sampling info"=w302, "formula"="a+a*f", "amplitude"=w319, "frequency"="Voltage step") -> ("signal out"=w315:waveform(dbl))  [unwired: 6 in, 1 out]
                n231 = local write "Frequency waveform"(w316) -> ()
                n232 = local write "Frequency"(w316) -> ()
                n233 = local write "Array 3"(w308) -> ()
                n234 = call "Sample Compression11"("Signals"=w310) -> ("Maximum"=w317:dynamicdata)  [unwired: 8 in, 2 out]
                n235 = call "Sample Compression12"("Signals"=w313) -> ("Maximum"=w312:dynamicdata)  [unwired: 8 in, 2 out]
                n236 = call "Sample Compression4"("Signals"=w315) -> ("Maximum"=w314:dynamicdata)  [unwired: 8 in, 2 out]
                n237 = local write "ROCOF waveform"(w317) -> ()
                n238 = local write "ROCOF"(w317) -> ()
                n239 = local read "Phase unit"() -> (w303:u16)
                n240 = call "Elapsed Time"() -> ("Elapsed Time (s)"=w332:dbl)  [unwired: 12 in, 7 out]
                n241 = call "phasePlotWrap.vi"("Sampling info"=w302, "Phase unit"=w303, "Phase"=w304, "Nominal Frequency"=w305, "Frequency"=w306) -> ("yScaleMin"=w299:dbl, "yScaleMax"=w300:dbl, "Phase waveform"=w301:waveform(dbl))  [unwired: 4 in]
                n242 = Less Or Equal?(x=w332, y=0.95) -> (x <= y?=w330:bool)
                n243 = local write "Phase waveform"(w301) -> ()
                n244 = property on="Phase waveform" class="WFChart (strict)"("YScale.Maximum"=w300) -> ()  [unwired: 2 in, 2 out]
                n245 = property on="Phase waveform" class="WFChart (strict)"("YScale.Minimum"=w299) -> ()  [unwired: 2 in, 2 out]
                n246 = local write "Phase"(w301) -> ()
                n247 = case shown="False" w330 {
                  tunnel: [w335 w337] -> w318
                  tunnel: w312 -> [_ w337]
                  tunnel: w314 -> [w335 _]
                  tunnel: [w334 w336] -> w309
                  tunnel: w313 -> [_ w336]
                  tunnel: w315 -> [w334 _]
                  frame False {
                  }
                  frame True {
                  }
                }
                "Voltage" <- w318
                "Array" <- w309
                n248 = local write "Votlage waveform"(w318) -> ()
                n249 = call-poly <vilib>:"Get Waveform Time Array.vi"("waveform in"=w309) -> ("X array"=w327:timestamp[])  [unwired: 9 in, 1 out]
                n250 = To Double Precision Float(number=w327) -> (double precision float=w328:dbl[])
                n251 = local write "double precision float"(w328) -> ()
                n252 = call "Elapsed Time2"() -> ("Time has Elapsed"=w329:bool)  [unwired: 12 in, 7 out]
                n253 = Stop(stop? (T)=w329) -> ()
              }
              frame 2 {
                w369 = TRUE
                w392 = FALSE ("Visible")
                # "phase step"
                # "nominal frequency"
                # "input voltage"
                # "input frequency"
                # "because the compression remove half of the sample so the last 0.1s will turn to 0.05s, delay 1s will be 0.95s instead"
                # "initial phase"
                n254 = local read "Sampling info"() -> (w340:cluster{"Fs":dbl, "#s":dbl})
                n255 = call <vilib>:"Formula Waveform.vi"("sampling info"=w340, "formula"="a", "amplitude"=w380) -> ("signal out"=w363:waveform(dbl))  [unwired: 7 in, 1 out]
                n256 = call <vilib>:"Formula Waveform.vi"("sampling info"=w340, "formula"="a", "amplitude"=w358) -> ("signal out"=w355:waveform(dbl))  [unwired: 7 in, 1 out]
                n257 = call <vilib>:"Formula Waveform.vi"("sampling info"=w340, "formula"="a", "amplitude"=w339) -> ("signal out"=w338:waveform(dbl))  [unwired: 7 in, 1 out]
                n258 = local write "Array"(w363) -> ()
                n259 = call <vilib>:"Formula Waveform.vi"("sampling info"=w340, "formula"="a", "amplitude"=w362) -> ("signal out"=w344:waveform(dbl))  [unwired: 7 in, 1 out]
                n260 = call-poly <vilib>:"Get Waveform Time Array.vi"("waveform in"=w363) -> ("X array"=w388:timestamp[])  [unwired: 9 in, 1 out]
                n261 = call "Sample Compression14"("Signals"=w363) -> ("Maximum"=w373:dynamicdata)  [unwired: 8 in, 2 out]
                n262 = call <vilib>:"Formula Waveform.vi"("sampling info"=w340, "formula"="a", "amplitude"=w378) -> ("signal out"=w368:waveform(dbl))  [unwired: 7 in, 1 out]
                n263 = call <vilib>:"Formula Waveform.vi"("sampling info"=w340, "formula"="a+1*f", "amplitude"=w378, "frequency"="Phase step") -> ("signal out"=w375:waveform(dbl))  [unwired: 6 in, 1 out]
                n264 = To Double Precision Float(number=w388) -> (double precision float=w387:dbl[])
                n265 = call "Sample Compression18"("Signals"=w355) -> ("Maximum"=w356:dynamicdata)  [unwired: 8 in, 2 out]
                n266 = call "Sample Compression17"("Signals"=w344) -> ("Maximum"=w360:dynamicdata)  [unwired: 8 in, 2 out]
                n267 = call "Sample Compression48"("Signals"=w338) -> ()  [unwired: 8 in, 3 out]
                n268 = call "Sample Compression15"("Signals"=w375) -> ("Maximum"=w374:dynamicdata)  [unwired: 8 in, 2 out]
                n269 = local write "double precision float"(w387) -> ()
                n270 = call "Sample Compression41"("Signals"=w368) -> ("Maximum"=w376:dynamicdata)  [unwired: 8 in, 2 out]
                n271 = local write "Voltage"(w373) -> ()
                n272 = local write "Votlage waveform"(w373) -> ()
                n273 = call "Elapsed Time4"() -> ("Elapsed Time (s)"=w393:dbl)  [unwired: 12 in, 7 out]
                n274 = Less Or Equal?(x=w393, y=0.95) -> (x <= y?=w357:bool)
                n275 = case shown="False" w357 {
                  tunnel: [w405 w407] -> w347
                  tunnel: w376 -> [_ w407]
                  tunnel: w374 -> [w405 _]
                  tunnel: w368 -> [_ w406]
                  tunnel: [w404 w406] -> w365
                  tunnel: w375 -> [w404 _]
                  frame False {
                  }
                  frame True {
                  }
                }
                "Array 2" <- w365
                n276 = Subtract(1:w368, 2:w365) -> (0:w367:waveform(dbl))  [unwired: 1 in, 1 out]
                n277 = call "Derivative (dX/dt)"("Signals"=w367) -> ("Result"=w345:dynamicdata)  [unwired: 5 in, 1 out]
                n278 = local read "Phase unit"() -> (w346:u16)
                n279 = Add(1:w344, 2:w345) -> (0:w343:dynamicdata)  [unwired: 1 in, 1 out]
                n280 = case shown="0, Default" w346 {
                  tunnel: w347 -> [w394 w395]
                  tunnel: [w394 w395] -> w342
                  frame 0, Default {
                  }
                  frame 1 {
                  }
                }
                "Phase" <- w342
                n281 = call "Sample Compression13"("Signals"=w343) -> ("Maximum"=w349:dynamicdata)  [unwired: 6 in, 4 out]
                n282 = case shown="False" w357 {
                  tunnel: w344 -> [_ w403]
                  tunnel: w360 -> [_ w402]
                  tunnel: [w401 w403] -> w351
                  tunnel: [w400 w402] -> w350
                  tunnel: w343 -> [w401 _]
                  tunnel: w349 -> [w400 _]
                  frame False {
                  }
                  frame True {
                  }
                }
                n283 = call "Convert from Dynamic Data7"("Dynamic Data Type"=w351) -> ("Array"=w364:dbl[])  [unwired: 3 in]
                n284 = local write "Phase waveform"(w342) -> ()
                n285 = call "Derivative (dX/dt)"("Signals"=w351) -> ("Result"=w353:dynamicdata)  [unwired: 5 in, 1 out]
                n286 = call "Elapsed Time5"() -> ("Time has Elapsed"=w391:bool)  [unwired: 12 in, 7 out]
                n287 = call "Convert from Dynamic Data"("Dynamic Data Type"=w350) -> ("Scalar"=w386:dbl)  [unwired: 3 in]
                n288 = call "Sample Compression16"("Signals"=w353) -> ("Maximum"=w348:dynamicdata)  [unwired: 5 in, 5 out]
                n289 = case shown="False" w357 {
                  tunnel: w356 -> [_ w399]
                  tunnel: w355 -> [_ w398]
                  tunnel: [w397 w399] -> w354
                  tunnel: [w396 w398] -> w352
                  tunnel: w348 -> [w397 _]
                  tunnel: w353 -> [w396 _]
                  frame False {
                  }
                  frame True {
                  }
                }
                n290 = call "Convert from Dynamic Data8"("Dynamic Data Type"=w352) -> ("Array"=w366:dbl[])  [unwired: 3 in]
                n291 = call "Convert from Dynamic Data2"("Dynamic Data Type"=w354) -> ("Scalar"=w383:dbl)  [unwired: 3 in]
                n292 = In Range and Coerce(upper limit=5.0, x=w383, lower limit=-5.0) -> (coerced(x)=w370:dbl)  [unwired: 1 out]
                "ROCOF waveform 2" <- w370
                n293 = In Range and Coerce(upper limit=55.0, x=w386, lower limit=45.0) -> (coerced(x)=w371:dbl)  [unwired: 1 out]
                "Frequency waveform 2" <- w371
                n294 = Stop(stop? (T)=w391) -> ()
                n295 = local write "Frequency"(w371) -> ()
                n296 = local write "ROCOF"(w370) -> ()
              }
              frame 3 {
                w446 = TRUE
                w449 = FALSE ("Visible")
                n297 = call "Elapsed Time7"() -> ("Time has Elapsed"=w465:bool)  [unwired: 12 in, 7 out]
                n298 = local read "Sampling info"() -> (w417:cluster{"Fs":dbl, "#s":dbl})
                n299 = call <vilib>:"Formula Waveform.vi"("sampling info"=w417, "formula"="a", "amplitude"=w447) -> ("signal out"=w444:waveform(dbl))  [unwired: 7 in, 1 out]
                n300 = local write "Array"(w444) -> ()
                n301 = call "Sample Compression22"("Signals"=w444) -> ("Maximum"=w450:dynamicdata)  [unwired: 8 in, 2 out]
                n302 = call <vilib>:"Formula Waveform.vi"("sampling info"=w417, "formula"="a", "amplitude"=w456) -> ("signal out"=w454:waveform(dbl))  [unwired: 7 in, 1 out]
                n303 = call <vilib>:"Formula Waveform.vi"("sampling info"=w417, "formula"="a", "amplitude"=w440) -> ("signal out"=w452:waveform(dbl))  [unwired: 7 in, 1 out]
                n304 = Stop(stop? (T)=w465) -> ()
                n305 = call <vilib>:"Formula Waveform.vi"("sampling info"=w417, "formula"="a", "amplitude"=w461) -> ("signal out"=w442:waveform(dbl))  [unwired: 7 in, 1 out]
                n306 = local write "Voltage"(w450) -> ()
                n307 = local write "Votlage waveform"(w450) -> ()
                n308 = call "Sample Compression29"("Signals"=w452) -> ()  [unwired: 8 in, 3 out]
                n309 = call "Sample Compression26"("Signals"=w454) -> ("Maximum"=w453:dynamicdata)  [unwired: 8 in, 2 out]
                n310 = call "Sample Compression20"("Signals"=w442) -> ("Maximum"=w455:dynamicdata)  [unwired: 8 in, 2 out]
                n311 = call <vilib>:"Formula Waveform.vi"("sampling info"=w417, "formula"="a+1*f", "amplitude"=w461, "frequency"="Frequency step") -> ("signal out"=w441:waveform(dbl))  [unwired: 6 in, 1 out]
                n312 = call "Elapsed Time6"() -> ("Elapsed Time (s)"=w468:dbl)  [unwired: 12 in, 7 out]
                n313 = call "Sample Compression27"("Signals"=w441) -> ("Maximum"=w451:dynamicdata)  [unwired: 8 in, 2 out]
                n314 = Less Or Equal?(x=w468, y=0.3) -> (x <= y?=w429:bool)
                n315 = local read "Phase unit"() -> (w419:u16)
                n316 = case shown="0, Default" w419 {
                  tunnel: [361.0 ("amplitude") 6.283185307179586] -> w420
                  frame 0, Default {
                  }
                  frame 1 {
                  }
                }
                n317 = case shown="False" w429 {
                  tunnel: [w515 w517] -> w437
                  tunnel: w455 -> [_ w517]
                  tunnel: w451 -> [w515 _]
                  tunnel: [w514 w516] -> w436
                  tunnel: w442 -> [_ w516]
                  tunnel: w441 -> [w514 _]
                  frame False {
                  }
                  frame True {
                  }
                }
                "Frequency" <- w437
                "Array 3" <- w436
                n318 = Subtract(1:w442, 2:w436) -> (0:w434:waveform(dbl))  [unwired: 1 in, 1 out]
                n319 = call "Derivative (dX/dt)"("Signals"=w434) -> ("Result"=w433:dynamicdata)  [unwired: 5 in, 1 out]
                n320 = call "Sample Compression30"("Signals"=w433) -> ("Mean"=w432:dynamicdata)  [unwired: 8 in, 2 out]
                n321 = call "Convert from Dynamic Data5"("Dynamic Data Type"=w432) -> ("Scalar"=w467:dbl)  [unwired: 3 in]
                n322 = In Range and Coerce(upper limit=5.0, x=w467, lower limit=-5.0) -> (coerced(x)=w448:dbl)  [unwired: 1 out]
                n323 = call "Convert from Dynamic Data4"("Dynamic Data Type"=w433) -> ("Array"=w443:dbl[])  [unwired: 3 in]
                n324 = local write "ROCOF"(w448) -> ()
                n325 = local write "ROCOF waveform 2"(w448) -> ()
                n326 = call <vilib>:"Formula Waveform.vi"("sampling info"=w417, "formula"="a", "amplitude"=360.0) -> ("signal out"=w408:waveform(dbl))  [unwired: 7 in, 1 out]
                n327 = local write "Frequency waveform"(w437) -> ()
                n328 = call-poly <vilib>:"Get Waveform Time Array.vi"("waveform in"=w436) -> ("X array"=w458:timestamp[])  [unwired: 9 in, 1 out]
                n329 = local read "Phase unit"() -> (w424:u16)
                n330 = call "Sample Compression47"("Signals"=w408) -> ("Maximum"=w410:dynamicdata)  [unwired: 8 in, 2 out]
                n331 = To Double Precision Float(number=w458) -> (double precision float=w457:dbl[])
                n332 = Greater?(x="Frequency step", y=0.0) -> (0:w411:bool)
                n333 = case shown="False" w411 {
                  tunnel: w420 -> [w491 w493]
                  tunnel: [w492 w493] -> w416
                  frame False {
                    n334 = Negate(x=w491) -> (-x=w492:dbl)
                  }
                  frame True {
                  }
                }
                n335 = case shown="False" w411 {
                  tunnel: w410 -> [w471 w472]
                  tunnel: [w470 w472] -> w409
                  frame False {
                    n336 = Negate(x=w471) -> (-x=w470:dynamicdata)
                  }
                  frame True {
                  }
                }
                n337 = call "Integral (Sum[Xdt])"("Signals"=w434) -> ("Result"=w426:dynamicdata)  [unwired: 5 in, 1 out]
                n338 = call "Convert from Dynamic Data11"() -> ("Scalar"=w466:dbl)  [unwired: 4 in]
                n339 = case shown="1, Default" w424 {
                  tunnel: [360.0 6.283185307179586] -> w428
                  tunnel: [w501 w503] -> w427
                  frame 0 {
                    n340 = Negate(x=360.0) -> (-x=w501:dbl)
                  }
                  frame 1, Default {
                    n341 = Negate(x=6.283185307179586) -> (-x=w503:dbl)
                  }
                }
                n342 = local write "double precision float"(w457) -> ()
                n343 = In Range and Coerce(upper limit=w428, x=w466, lower limit=w427) -> (coerced(x)=→"Phase waveform 2":dbl)  [unwired: 1 out]
                n344 = case shown="1" w424 {
                  tunnel: w426 -> [w495 w498]
                  tunnel: [w494 w497] -> w425
                  frame 0, Default {
                    n345 = Multiply(x=w495, y=360.0) -> (x*y=w494:dynamicdata)
                  }
                  frame 1 {
                    n346 = Multiply(x=w498, y=6.283185307179586) -> (x*y=w497:dynamicdata)
                  }
                }
                n347 = call "Sample Compression19"("Signals"=w425) -> ("Maximum"=w431:dynamicdata)  [unwired: 8 in, 2 out]
                n348 = case shown="False" w429 {
                  tunnel: [w510 w513] -> w414
                  tunnel: w453 -> [_ w513]
                  tunnel: w425 -> [w511 _]
                  tunnel: w454 -> [_ w512]
                  tunnel: [w511 w512] -> w430
                  tunnel: w431 -> [w510 _]
                  frame False {
                  }
                  frame True {
                  }
                }
                n349 = call "Convert from Dynamic Data6"("Dynamic Data Type"=w430) -> ("Array"=w435:dbl[])  [unwired: 3 in]
                n350 = case shown="False" w429 {
                  tunnel: [w507 w509] -> _
                  tunnel: w453 -> [w507 w508]
                  tunnel: [w506 w508] -> w445
                  tunnel: w454 -> [w506 _]
                  tunnel: w414 -> [_ w509]
                  frame False {
                  }
                  frame True {
                  }
                }
                n351 = for {
                  N: 50 -> [_]
                  tunnel: w416 -> [w477]
                  shift-right: [w474] -> w412
                  shift-left: w414 -> [w475]
                  tunnel: w409 -> [w476]
                  tunnel: w411 -> [w473]
                  n352 = case shown="True" w473 {
                    tunnel: w475 -> [w481 w484]
                    tunnel: [w480 w483] -> w478
                    tunnel: w477 -> [w479 w482]
                    frame False {
                      n353 = Less Or Equal?(x=w481, y=w479) -> (x <= y?=w480:dynamicdata)
                    }
                    frame True {
                      n354 = Greater Or Equal?(x=w484, y=w482) -> (x >= y?=w483:dynamicdata)
                    }
                  }
                  n355 = case shown="True" w478 {
                    tunnel: w475 -> [w485 w488]
                    tunnel: [w485 w486] -> w474
                    tunnel: w476 -> [_ w487]
                    frame False {
                    }
                    frame True {
                      n356 = Subtract(1:w487, 2:w488) -> (0:w486:dynamicdata)  [unwired: 1 in, 1 out]
                    }
                  }
                }
                n357 = local write "Array 2"(w445) -> ()
                n358 = local write "Phase waveform"(w412) -> ()
                n359 = local write "Phase"(w412) -> ()
              }
              frame 4 {
                w579 = TRUE ("Visible")
                w546 = FALSE ("Visible")
                n360 = local read "Phase unit"() -> (w531:u16)
                n361 = local read "Sampling info"() -> (w548:cluster{"Fs":dbl, "#s":dbl})
                n362 = case shown="0, Default" w531 {
                  tunnel: [365.0 ("amplitude") 6.283185307179586] -> w530
                  frame 0, Default {
                  }
                  frame 1 {
                  }
                }
                n363 = call <vilib>:"Formula Waveform.vi"("sampling info"=w548, "formula"="a", "amplitude"="ROCOF rate") -> ("signal out"=w566:waveform(dbl))  [unwired: 7 in, 1 out]
                n364 = local read "Sampling info"() -> (w547:cluster{"Fs":dbl, "#s":dbl})
                n365 = call "Sample Compression36"("Signals"=w566) -> ()  [unwired: 8 in, 3 out]
                n366 = call <vilib>:"Formula Waveform.vi"("sampling info"=w547, "formula"="a", "amplitude"=w550) -> ("signal out"=w544:waveform(dbl))  [unwired: 7 in, 1 out]
                n367 = call <vilib>:"Formula Waveform.vi"("sampling info"=w548, "formula"="a", "amplitude"=w545) -> ("signal out"=w535:waveform(dbl))  [unwired: 7 in, 1 out]
                n368 = call <vilib>:"Formula Waveform.vi"("sampling info"=w548, "formula"="a", "amplitude"=w563) -> ("signal out"=w560:waveform(dbl))  [unwired: 7 in, 1 out]
                n369 = call <vilib>:"Formula Waveform.vi"("sampling info"=w548, "formula"="a", "amplitude"=360.0) -> ("signal out"=w527:waveform(dbl))  [unwired: 7 in, 1 out]
                n370 = call "Sample Compression32"("Signals"=w544) -> ("Maximum"=w549:dynamicdata)  [unwired: 8 in, 2 out]
                n371 = local write "Array"(w544) -> ()
                n372 = call "Elapsed Time10"() -> ("Elapsed Time (s)"=w577:dbl)  [unwired: 12 in, 7 out]
                n373 = call "Sample Compression37"("Signals"=w560) -> ("Maximum"=w561:dynamicdata)  [unwired: 8 in, 2 out]
                n374 = call "Sample Compression40"("Signals"=w527) -> ("Maximum"=w519:dynamicdata)  [unwired: 8 in, 2 out]
                n375 = call "Sample Compression34"("Signals"=w535) -> ("Maximum"=w568:dynamicdata)  [unwired: 8 in, 2 out]
                n376 = Less Or Equal?(x=w577, y=0.3) -> (x <= y?=w564:bool)
                n377 = Greater?(x="ROCOF rate", y=0.0) -> (0:w558:bool)
                n378 = local write "Votlage waveform"(w549) -> ()
                n379 = local write "Voltage"(w549) -> ()
                n380 = call <vilib>:"Formula Waveform.vi"("sampling info"=w548, "formula"="a", "amplitude"="Final freq.") -> ("signal out"=w536:waveform(dbl))  [unwired: 7 in, 1 out]
                n381 = call "Sample Compression33"("Signals"=w536) -> ("Maximum"=w573:dynamicdata)  [unwired: 8 in, 2 out]
                n382 = Greater?(x="ROCOF rate", y=0.0) -> (0:w520:bool)
                n383 = case shown="False" w520 {
                  tunnel: w530 -> [w605 w607]
                  tunnel: [w606 w607] -> w524
                  frame False {
                    n384 = Negate(x=w605) -> (-x=w606:dbl)
                  }
                  frame True {
                  }
                }
                n385 = call <vilib>:"Formula Waveform.vi"("sampling info"=w548, "formula"="(a-0.3*f)+f*t", "amplitude"=w545, "frequency"="ROCOF rate") -> ("signal out"=w553:waveform(dbl))  [unwired: 6 in, 1 out]
                n386 = call "Sample Compression31"("Signals"=w553) -> ("Maximum"=w552:dynamicdata)  [unwired: 8 in, 2 out]
                n387 = case shown="False" w558 {
                  tunnel: w552 -> [w610 w613]
                  tunnel: "Final freq." -> [w609 w612]
                  tunnel: [w608 w611] -> w556
                  frame False {
                    n388 = Greater?(x=w610, y=w609) -> (0:w608:dynamicdata)
                  }
                  frame True {
                    n389 = Less?(x=w613, y=w612) -> (x < y?=w611:dynamicdata)
                  }
                }
                n390 = case shown="False" w564 {
                  tunnel: w568 -> [_ w621]
                  tunnel: w535 -> [_ w620]
                  tunnel: [w619 w621] -> w571
                  tunnel: [w618 w620] -> w537
                  tunnel: w552 -> [w619 _]
                  tunnel: w553 -> [w618 _]
                  frame False {
                  }
                  frame True {
                  }
                }
                n391 = case shown="True" w556 {
                  tunnel: [w623 w625] -> w543
                  tunnel: w573 -> [w623 _]
                  tunnel: [w622 w624] -> w542
                  tunnel: w536 -> [w622 _]
                  tunnel: w571 -> [_ w625]
                  tunnel: w537 -> [_ w624]
                  frame False {
                  }
                  frame True {
                  }
                }
                n392 = case shown="False" w520 {
                  tunnel: w519 -> [w581 w582]
                  tunnel: [w580 w582] -> w518
                  frame False {
                    n393 = Negate(x=w581) -> (-x=w580:dynamicdata)
                  }
                  frame True {
                  }
                }
                n394 = local read "Phase unit"() -> (w534:u16)
                n395 = Subtract(1:w535, 2:w542) -> (0:w541:waveform(dbl))  [unwired: 1 in, 1 out]
                n396 = call "Integral (Sum[Xdt])"("Signals"=w541) -> ("Result"=w533:dynamicdata)  [unwired: 5 in, 1 out]
                n397 = case shown="0, Default" w534 {
                  tunnel: w533 -> [w603 w604]
                  tunnel: [w601 w604] -> w532
                  frame 0, Default {
                    n398 = Multiply(x=w603, y=360.0) -> (x*y=w601:dynamicdata)
                  }
                  frame 1 {
                  }
                }
                n399 = call-poly <vilib>:"Get Waveform Time Array.vi"("waveform in"=w542) -> ("X array"=w570:timestamp[])  [unwired: 9 in, 1 out]
                n400 = local write "Frequency waveform"(w543) -> ()
                n401 = local write "Array 3"(w542) -> ()
                n402 = local write "Frequency"(w543) -> ()
                n403 = call "Derivative (dX/dt)"("Signals"=w541) -> ("Result"=w529:dynamicdata)  [unwired: 5 in, 1 out]
                n404 = call "Convert from Dynamic Data12"("Dynamic Data Type"=w529) -> ("Array"=w528:dbl[])  [unwired: 3 in]
                n405 = To Double Precision Float(number=w570) -> (double precision float=w569:dbl[])
                n406 = local write "double precision float"(w569) -> ()
                n407 = call "Elapsed Time8"() -> ("Time has Elapsed"=w576:bool)  [unwired: 12 in, 7 out]
                n408 = call "Sample Compression28"("Signals"=w529) -> ("Maximum"=w521:dynamicdata)  [unwired: 8 in, 2 out]
                n409 = call "Sample Compression39"("Signals"=w532) -> ("Maximum"=w540:dynamicdata)  [unwired: 8 in, 2 out]
                n410 = case shown="False" w564 {
                  tunnel: w561 -> [_ w617]
                  tunnel: [w615 w617] -> w525
                  tunnel: w560 -> [_ w616]
                  tunnel: [w614 w616] -> w538
                  tunnel: w540 -> [w615 _]
                  tunnel: w532 -> [w614 _]
                  frame False {
                  }
                  frame True {
                  }
                }
                n411 = call "Convert from Dynamic Data9"("Dynamic Data Type"=w538) -> ("Array"=w539:dbl[])  [unwired: 3 in]
                n412 = for {
                  N: 50 -> [_]
                  tunnel: w524 -> [w587]
                  shift-right: [w584] -> w523
                  shift-left: w525 -> [w585]
                  tunnel: w518 -> [w586]
                  tunnel: w520 -> [w583]
                  n413 = case shown="True" w583 {
                    tunnel: w585 -> [w591 w594]
                    tunnel: [w590 w593] -> w588
                    tunnel: w587 -> [w589 w592]
                    frame False {
                      n414 = Less Or Equal?(x=w591, y=w589) -> (x <= y?=w590:dynamicdata)
                    }
                    frame True {
                      n415 = Greater?(x=w594, y=w592) -> (0:w593:dynamicdata)
                    }
                  }
                  n416 = case shown="True" w588 {
                    tunnel: w585 -> [w595 w598]
                    tunnel: [w595 w596] -> w584
                    tunnel: w586 -> [_ w597]
                    frame False {
                    }
                    frame True {
                      n417 = Subtract(1:w597, 2:w598) -> (0:w596:dynamicdata)  [unwired: 1 in, 1 out]
                    }
                  }
                }
                n418 = Stop(stop? (T)=w576) -> ()
                n419 = local write "ROCOF waveform"(w521) -> ()
                n420 = local write "ROCOF"(w521) -> ()
                n421 = local write "Phase waveform"(w523) -> ()
                n422 = local write "Phase"(w523) -> ()
              }
              frame 5 {
                w659 = TRUE
                w634 = FALSE
                n423 = call "Elapsed Time11"() -> ("Elapsed Time (s)"=w658:dbl)  [unwired: 12 in, 7 out]
                n424 = Less Or Equal?(x=w658, y=0.3) -> (x <= y?=w656:bool)
                n425 = call <vilib>:"Formula Waveform.vi"("sampling info"="Sampling info", "formula"="a", "amplitude"=w648) -> ("signal out"=w632:waveform(dbl))  [unwired: 7 in, 1 out]
                n426 = call <vilib>:"Formula Waveform.vi"("sampling info"="Sampling info", "formula"="a", "amplitude"=w651) -> ("signal out"=w630:waveform(dbl))  [unwired: 7 in, 1 out]
                n427 = call <vilib>:"Formula Waveform.vi"("sampling info"="Sampling info", "formula"="a", "amplitude"=w647) -> ("signal out"=w631:waveform(dbl))  [unwired: 7 in, 1 out]
                n428 = local write "Array 2"(w630) -> ()
                n429 = call "Sample Compression"("Signals"=w630) -> ("Maximum"=w627:dynamicdata)  [unwired: 8 in, 2 out]
                n430 = local write "Array 3"(w632) -> ()
                n431 = call "Sample Compression23"("Signals"=w632) -> ("Maximum"=w633:dynamicdata)  [unwired: 8 in, 2 out]
                n432 = call "Sample Compression24"("Signals"=w631) -> ("Maximum"=w646:dynamicdata)  [unwired: 8 in, 2 out]
                n433 = call <vilib>:"Formula Waveform.vi"("sampling info"="Sampling info", "formula"="a", "amplitude"=w636) -> ("signal out"=w640:waveform(dbl))  [unwired: 7 in, 1 out]
                n434 = local read "Phase unit"() -> (w628:u16)
                n435 = call <vilib>:"Formula Waveform.vi"("offset"=w636, "sampling info"="Sampling info", "formula"="a*sin(2*pi(1)*f*t)", "amplitude"="Mod Amp", "frequency"="Mod Freq") -> ("signal out"=w641:waveform(dbl))  [unwired: 5 in, 1 out]
                n436 = local write "Frequency waveform"(w633) -> ()
                n437 = local write "ROCOF waveform"(w646) -> ()
                n438 = call "Sample Compression21"("Signals"=w641) -> ("Maximum"=w638:dynamicdata)  [unwired: 8 in, 2 out]
                n439 = call "Sample Compression43"("Signals"=w640) -> ("Maximum"=w639:dynamicdata)  [unwired: 8 in, 2 out]
                n440 = case shown="True" w656 {
                  tunnel: w636 -> [_ _]
                  tunnel: [w667 w669] -> w629
                  tunnel: w640 -> [_ w669]
                  tunnel: w641 -> [w667 _]
                  tunnel: w639 -> [_ w668]
                  tunnel: [w666 w668] -> w637
                  tunnel: w638 -> [w666 _]
                  frame False {
                  }
                  frame True {
                  }
                }
                n441 = case shown="1" w628 {
                  tunnel: w627 -> [w664 w665]
                  tunnel: [w660 w665] -> w626
                  frame 0, Default {
                    n442 = Multiply(x=w664, y=180.0) -> (x*y=w661:dynamicdata)
                    n443 = Divide(x=w661, y=3.141592653589793) -> (x/y=w660:dynamicdata)
                  }
                  frame 1 {
                  }
                }
                n444 = local write "Phase"(w627) -> ()
                n445 = local write "Frequency"(w633) -> ()
                n446 = local write "ROCOF"(w646) -> ()
                n447 = local write "Phase waveform"(w626) -> ()
                n448 = local write "Votlage waveform"(w637) -> ()
                n449 = local write "Array"(w629) -> ()
                n450 = call-poly <vilib>:"Get Waveform Time Array.vi"("waveform in"=w630) -> ("X array"=w654:timestamp[])  [unwired: 9 in, 1 out]
                n451 = local write "Voltage"(w629) -> ()
                n452 = To Double Precision Float(number=w654) -> (double precision float=w653:dbl[])
                n453 = local write "double precision float"(w653) -> ()
                n454 = call "Elapsed Time9"() -> ("Time has Elapsed"=w655:bool)  [unwired: 12 in, 7 out]
                n455 = Stop(stop? (T)=w655) -> ()
              }
              frame 6 {
                w713 = TRUE
                w680 = FALSE
                n456 = call "Elapsed Time12"() -> ("Elapsed Time (s)"=w711:dbl)  [unwired: 12 in, 7 out]
                n457 = local read "Sampling info"() -> (w684:cluster{"Fs":dbl, "#s":dbl})
                n458 = Less Or Equal?(x=w711, y=0.3) -> (x <= y?=w701:bool)
                n459 = call <vilib>:"Formula Waveform.vi"("sampling info"=w684, "formula"="a", "amplitude"=w707) -> ("signal out"=w673:waveform(dbl))  [unwired: 7 in, 1 out]
                n460 = call "Sample Compression25"("Signals"=w673) -> ("Maximum"=w706:dynamicdata)  [unwired: 8 in, 2 out]
                n461 = Multiply(x="Mod Amp", y="Mod Freq") -> (x*y=→"Freq Dev":dbl)
                n462 = call <vilib>:"Formula Waveform.vi"("sampling info"=w684, "formula"="a", "amplitude"=w682) -> ("signal out"=w698:waveform(dbl))  [unwired: 7 in, 1 out]
                n463 = call <vilib>:"Formula Waveform.vi"("offset"=w682, "sampling info"=w684, "formula"="a*cos(2*pi(1)*f*t-pi(1))", "amplitude"="Mod Amp", "frequency"="Mod Freq") -> ("signal out"=w697:waveform(dbl))  [unwired: 5 in, 1 out]
                n464 = call <vilib>:"Formula Waveform.vi"("offset"=w683, "sampling info"=w684, "formula"="-a*f*sin(2*pi(1)*f*t-pi(1))", "amplitude"="Mod Amp", "frequency"="Mod Freq") -> ("signal out"=w693:waveform(dbl))  [unwired: 5 in, 1 out]
                n465 = call <vilib>:"Formula Waveform.vi"("sampling info"=w684, "formula"="a", "amplitude"=w683) -> ("signal out"=w694:waveform(dbl))  [unwired: 7 in, 1 out]
                n466 = call <vilib>:"Formula Waveform.vi"("sampling info"=w684, "formula"="a", "amplitude"=w681) -> ("signal out"=w689:waveform(dbl))  [unwired: 7 in, 1 out]
                n467 = call <vilib>:"Formula Waveform.vi"("offset"=w681, "sampling info"=w684, "formula"="-a*2*pi(1)*f*f*cos(2*pi(1)*f*t-pi(1))", "amplitude"="Mod Amp", "frequency"="Mod Freq") -> ("signal out"=w688:waveform(dbl))  [unwired: 5 in, 1 out]
                n468 = local write "Array"(w673) -> ()
                n469 = local write "Voltage"(w706) -> ()
                n470 = call "Sample Compression2"("Signals"=w698) -> ("Maximum"=w696:dynamicdata)  [unwired: 8 in, 2 out]
                n471 = call "Sample Compression42"("Signals"=w694) -> ("Maximum"=w691:dynamicdata)  [unwired: 8 in, 2 out]
                n472 = call "Sample Compression44"("Signals"=w689) -> ("Maximum"=w686:dynamicdata)  [unwired: 8 in, 2 out]
                n473 = call-poly <vilib>:"Get Waveform Time Array.vi"("waveform in"=w673) -> ("X array"=w710:timestamp[])  [unwired: 9 in, 1 out]
                n474 = local write "Votlage waveform"(w706) -> ()
                n475 = To Double Precision Float(number=w710) -> (double precision float=w709:dbl[])
                n476 = call "Sample Compression45"("Signals"=w697) -> ("Maximum"=w695:dynamicdata)  [unwired: 8 in, 2 out]
                n477 = case shown="False" w701 {
                  tunnel: [w730 w732] -> w676
                  tunnel: w698 -> [_ w732]
                  tunnel: w697 -> [w730 _]
                  tunnel: [w729 w731] -> w671
                  tunnel: w696 -> [_ w731]
                  tunnel: w695 -> [w729 _]
                  frame False {
                  }
                  frame True {
                  }
                }
                n478 = call "Sample Compression46"("Signals"=w693) -> ("Maximum"=w692:dynamicdata)  [unwired: 8 in, 2 out]
                n479 = case shown="True" w701 {
                  tunnel: [w726 w728] -> w674
                  tunnel: w694 -> [_ w728]
                  tunnel: w693 -> [w726 _]
                  tunnel: [w725 w727] -> w690
                  tunnel: w692 -> [w725 _]
                  tunnel: w691 -> [_ w727]
                  frame False {
                  }
                  frame True {
                  }
                }
                n480 = local write "double precision float"(w709) -> ()
                n481 = call "Sample Compression3"("Signals"=w688) -> ("Maximum"=w687:dynamicdata)  [unwired: 8 in, 2 out]
                n482 = case shown="True" w701 {
                  tunnel: [w722 w724] -> w675
                  tunnel: w689 -> [_ w724]
                  tunnel: w688 -> [w722 _]
                  tunnel: [w721 w723] -> w685
                  tunnel: w687 -> [w721 _]
                  tunnel: w686 -> [_ w723]
                  frame False {
                  }
                  frame True {
                  }
                }
                n483 = local read "Phase unit"() -> (w672:u16)
                n484 = case shown="0, Default" w672 {
                  tunnel: w671 -> [w719 w720]
                  tunnel: [w715 w720] -> w670
                  frame 0, Default {
                    n485 = Multiply(x=w719, y=180.0) -> (x*y=w716:dynamicdata)
                    n486 = Divide(x=w716, y=3.141592653589793) -> (x/y=w715:dynamicdata)
                  }
                  frame 1 {
                  }
                }
                n487 = local write "Frequency waveform"(w690) -> ()
                n488 = local write "Array 2"(w676) -> ()
                n489 = local write "Phase"(w676) -> ()
                n490 = local write "ROCOF"(w675) -> ()
                n491 = local write "ROCOF waveform"(w685) -> ()
                n492 = local write "Frequency"(w674) -> ()
                n493 = local write "Array 3"(w674) -> ()
                n494 = local write "Phase waveform"(w670) -> ()
                n495 = call "Elapsed Time13"() -> ("Time has Elapsed"=w712:bool)  [unwired: 12 in, 7 out]
                n496 = Stop(stop? (T)=w712) -> ()
              }
              frame 7 {
                w733 = dbl[] []
                w734 = FALSE
                w736 = TRUE
                n497 = local write "Voltage"(w735) -> ()
                n498 = local write "Frequency"(w737) -> ()
              }
            }
          }
        }
        n499 = case shown="True" w166 {
          tunnel: [w180 w204] -> w172
          tunnel: [w181 w197] -> w171
          tunnel: w174 -> [w181 w188]
          tunnel: w173 -> [w180 w187]
          tunnel: w169 -> [_ w185]
          tunnel: w170 -> [_ w184]
          tunnel: w168 -> [_ w183]
          tunnel: w167 -> [_ w182]
          frame False {
          }
          frame True {
            w189 = "3 Phase Generator" ("group name in (Untitled)")
            n500 = local read "double precision float"() -> (w186:dbl[])
            n501 = Build Array(w184) -> (w200:dbl[][])
            n502 = Build Array(w183) -> (w199:dbl[][])
            n503 = Build Array(w182) -> (w198:dbl[][])
            n504 = Build Array(w185) -> (w208:dbl[][])
            n505 = TDMS Write(0:w188, 5:w189, 7:"Time" ("channel name(s) in (Untitled)"), 9:w186, 11:w187) -> (4:w192:refnum<k34>, 15:w191:errorcluster)  [unwired: 1 in, 2 out]
            n506 = TDMS Write(0:w192, 5:w189, 7:string[] ["Voltage"] ("channel name(s) in (Untitled)"), 9:w208, 11:w191) -> (4:w203:refnum<k34>, 15:w207:errorcluster)  [unwired: 1 in, 2 out]
            n507 = TDMS Write(0:w203, 5:w189, 7:string[] ["Phase"] ("channel name(s) in (Untitled)"), 9:w200, 11:w207) -> (4:w202:refnum<k34>, 15:w206:errorcluster)  [unwired: 1 in, 2 out]
            n508 = TDMS Write(0:w202, 5:w189, 7:string[] ["Frequency"] ("channel name(s) in (Untitled)"), 9:w199, 11:w206) -> (4:w201:refnum<k34>, 15:w205:errorcluster)  [unwired: 1 in, 2 out]
            n509 = TDMS Write(0:w201, 5:w189, 7:string[] ["ROCOF"] ("channel name(s) in (Untitled)"), 9:w198, 11:w205) -> (4:w197:refnum<k34>, 15:w204:errorcluster)  [unwired: 1 in, 2 out]
          }
        }
        n510 = property on="Mod Freq" class="DigNum (strict)"("Visible"=w161) -> ()  [unwired: 2 in, 2 out]
        n511 = property on="Initial freq." class="DigNum (strict)"("Visible"=w159) -> ()  [unwired: 2 in, 2 out]
        n512 = property on="FreqDev" class="Str"("Visible"=w161) -> ()  [unwired: 2 in, 2 out]
        n513 = property on="Final freq." class="DigNum (strict)"("Visible"=w159) -> ()  [unwired: 2 in, 2 out]
        n514 = property on="Phase waveform 2" class="WFChart (strict)"("Visible"=w164) -> ()  [unwired: 2 in, 2 out]
        n515 = property on="H2 order" class="DigNum (strict)"("Visible"=w164) -> ()  [unwired: 2 in, 2 out]
        n516 = property on="Freq Dev" class="DigNum (strict)"("Visible"=w161) -> ()  [unwired: 2 in, 2 out]
        n517 = property on="H2 Volt" class="DigNum (strict)"("Visible"=w164) -> ()  [unwired: 2 in, 2 out]
        n518 = property on="H2 Phase" class="DigNum (strict)"("Visible"=w164) -> ()  [unwired: 2 in, 2 out]
        n519 = property on="H1 order" class="DigNum (strict)"("Visible"=w164) -> ()  [unwired: 2 in, 2 out]
        n520 = property on="H1 Phase" class="DigNum (strict)"("Visible"=w164) -> ()  [unwired: 2 in, 2 out]
        n521 = property on="Mod Freq" class="DigNum (strict)"("Visible"=w162) -> ()  [unwired: 2 in, 2 out]
        n522 = property on="H1 Volt" class="DigNum (strict)"("Visible"=w164) -> ()  [unwired: 2 in, 2 out]
        n523 = property on="ROCOF rate" class="DigNum (strict)"("Visible"=w159) -> ()  [unwired: 2 in, 2 out]
        n524 = property on="ROCOF waveform 2" class="WFChart (strict)"("Visible"=w175) -> ()  [unwired: 2 in, 2 out]
        n525 = property class="Str"("Visible"=w162) -> ()  [unwired: 2 in, 2 out]
        n526 = property on="Phase step" class="DigNum (strict)"("Visible"=w163) -> ()  [unwired: 2 in, 2 out]
        n527 = property on="Frequency" class="DigNum (strict)"("Visible"=w176) -> ()  [unwired: 2 in, 2 out]
        n528 = property on="2" class="WFChart (strict)"("Visible"=w177) -> ()  [unwired: 2 in, 2 out]
        n529 = property on="Mod Amp" class="DigNum (strict)"("Visible"=w161) -> ()  [unwired: 2 in, 2 out]
        n530 = property on="Mod Amp" class="DigNum (strict)"("Visible"=w162) -> ()  [unwired: 2 in, 2 out]
        n531 = property on="PMFeq" class="Str"("Visible"=w161) -> ()  [unwired: 2 in, 2 out]
        n532 = property on="Time" class="DigNum (strict)"("Visible"=w159) -> ()  [unwired: 2 in, 2 out]
        n533 = property on="second" class="Str"("Visible"=w159) -> ()  [unwired: 2 in, 2 out]
        n534 = property on="Final freq" class="Str"("Visible"=w159) -> ()  [unwired: 2 in, 2 out]
        n535 = property on="Hz/s" class="Str"("Visible"=w159) -> ()  [unwired: 2 in, 2 out]
        n536 = property on="Voltage step" class="DigNum (strict)"("Visible"=w158) -> ()  [unwired: 2 in, 2 out]
        n537 = property on="Frequency step" class="DigNum (strict)"("Visible"=w165) -> ()  [unwired: 2 in, 2 out]
        n538 = property class="Str"("Visible"=w165) -> ()  [unwired: 2 in, 2 out]
      }
      frame #3 {
        n539 = case shown="True" w738 {
          frame False {
          }
          frame True {
            w827 = u8 0  # U8
            # "calculations are done in radian but phasor uses degree so convert rad to deg"
            n540 = local read "Select test type"() -> (w830:u16)
            n541 = case shown="0, Default" w830 {
              tunnel: [0 1 2 3 4 5 6 7] -> w779
              tunnel: [w853 w862 w874 w896 w929 w950 w968 w991] -> w804
              tunnel: [w852 w861 w873 w895 w928 w949 w967 w972] -> w810
              tunnel: [w851 w860 w872 w894 w927 w948 w966 w990] -> w829
              tunnel: [w850 w856 w865 w887 w919 w945 w963 w989] -> w778
              tunnel: [w850 w855 w864 w893 w909 w930 w952 w983] -> w776
              tunnel: [w850 w855 w864 w893 w913 w943 w953 w993] -> w774
              tunnel: [w850 w855 w864 w893 w913 w930 w952 w978] -> w772
              frame 0, Default {
                w850 = 0.0
                n542 = local read "Frequency"() -> (w851:dbl)
                n543 = local read "Phase"() -> (w852:dbl)
                n544 = local read "Voltage"() -> (w853:dbl)
              }
              frame 1 {
                w855 = 0.0
                n545 = local read "Voltage"() -> (w857:dbl)
                n546 = local read "Phase"() -> (w861:dbl)
                n547 = local read "Frequency"() -> (w860:dbl)
                n548 = local read "Voltage"() -> (w862:dbl)
                n549 = Multiply(x=w857, y=52428.8) -> (x*y=w859:dbl)
                n550 = Round Toward +Infinity(x=w859) -> (ceil(x): smallest int >= x=w856:dbl)
              }
              frame 2 {
                w864 = 0.0
                n551 = local read "Phase"() -> (w866:dbl)
                n552 = local read "Phase"() -> (w873:dbl)
                n553 = Divide(x=w866, y=360.0) -> (x/y=w868:dbl)
                n554 = local read "Frequency"() -> (w872:dbl)
                n555 = Power Of X(1:2.0 ("x"), 2:16.0 ("y")) -> (0:w867:dbl)
                n556 = local read "Voltage"() -> (w874:dbl)
                n557 = Multiply(x=w867, y=w868) -> (x*y=w865:dbl)
              }
              frame 3 {
                w893 = 0.0
                n558 = local read "Frequency"() -> (w877:dbl)
                n559 = Power Of X(1:2.0 ("x"), 2:31.0 ("y")) -> (0:w882:dbl)
                n560 = local read "Phase"() -> (w895:dbl)
                n561 = local read "Frequency"() -> (w894:dbl)
                n562 = Power Of X(1:10.0 ("x"), 2:6.0 ("y")) -> (0:w884:dbl)
                n563 = local read "Voltage"() -> (w896:dbl)
                n564 = Multiply(x=w877, y=w882) -> (x*y=w885:dbl)
                n565 = Multiply(x=2.5, y=w884) -> (x*y=w886:dbl)
                n566 = Divide(x=w885, y=w886) -> (x/y=w876:dbl)
                n567 = Round Toward +Infinity(x=w876) -> (ceil(x): smallest int >= x=w892:dbl)
                n568 = Number To Hexadecimal String(2:w892) -> (0:w891:string)  [unwired: 1 in]
                n569 = String Subset(string=w891, offset (0)=0, length (rest)=4 ("length (rest)")) -> (substring=w888:string)
                n570 = Hexadecimal String To Number(string=w888) -> (number=w887:u32)  [unwired: 2 in, 1 out]
              }
              frame 4 {
                w913 = 0.0
                n571 = local read "Final freq."() -> (w906:dbl)
                n572 = local read "ROCOF rate"() -> (w904:dbl)
                n573 = local read "Frequency"() -> (w898:dbl)
                n574 = Power Of X(1:10.0 ("x"), 2:6.0 ("y")) -> (0:w917:dbl)
                n575 = Power Of X(1:2.0 ("x"), 2:42.0 ("y")) -> (0:w922:dbl)
                n576 = local read "Frequency"() -> (w927:dbl)
                n577 = local read "Phase"() -> (w928:dbl)
                n578 = Subtract(x=w906, y=w898) -> (x-y=w905:dbl)
                n579 = local read "Voltage"() -> (w929:dbl)
                n580 = Divide(x=2500000.0, y=64.0) -> (x/y=w923:dbl)
                n581 = Multiply(x=w905, y=w904) -> (x*y=w903:dbl)
                "Time" <- w903
                n582 = Multiply(x=w903, y=w917) -> (x*y=w914:dbl)
                n583 = Multiply(x=2.5, y=w914) -> (x*y=w900:dbl)
                n584 = Multiply(x=w904, y=w922) -> (x*y=w921:dbl)
                n585 = Square(x=w923) -> (x^2=w920:dbl)
                n586 = Divide(x=w900, y=1024.0) -> (x/y=w899:dbl)
                n587 = Number To Hexadecimal String(2:w899) -> (0:w911:string)  [unwired: 1 in]
                n588 = Divide(x=w921, y=w920) -> (x/y=w919:dbl)
                n589 = String Subset(string=w911, offset (0)=0, length (rest)=4 ("length (rest)")) -> (substring=w910:string)
                n590 = Hexadecimal String To Number(string=w910) -> (number=w909:u32)  [unwired: 2 in, 1 out]
              }
              frame 5 {
                w930 = 0.0 ("Frequency")
                n591 = local read "Mod Amp"() -> (w947:dbl)
                n592 = local read "Mod Freq"() -> (w935:dbl)
                n593 = local read "Phase"() -> (w949:dbl)
                n594 = local read "Frequency"() -> (w948:dbl)
                n595 = local read "Voltage"() -> (w950:dbl)
                n596 = Multiply(x=w935, y=68719476736.0) -> (x*y=w932:dbl)
                n597 = Divide(x=w932, y=2500000.0) -> (x/y=w931:dbl)
                n598 = Multiply(x=w947, y=41943.04) -> (x*y=w938:dbl)
                n599 = Multiply(x=10.0, y=w938) -> (x*y=w937:dbl)
                n600 = Format Into String(format string="%4x", w931) -> (resulting string=w942:string)  [unwired: 2 in, 1 out]
                n601 = Round Toward -Infinity(1:w937) -> (0:w945:dbl)
                n602 = String Subset(string=w942, offset (0)=0, length (rest)=4 ("length (rest)")) -> (substring=w939:string)
                n603 = Hexadecimal String To Number(string=w939) -> (number=w943:u32)  [unwired: 2 in, 1 out]
              }
              frame 6 {
                w952 = 0.0
                n604 = local read "Mod Freq"() -> (w957:dbl)
                n605 = local read "Mod Amp"() -> (w964:dbl)
                n606 = local read "Phase"() -> (w967:dbl)
                n607 = local read "Frequency"() -> (w966:dbl)
                n608 = local read "Voltage"() -> (w968:dbl)
                n609 = Multiply(x=w957, y=68719476736.0) -> (x*y=w954:dbl)
                n610 = Divide(x=w954, y=2500000.0) -> (x/y=w953:dbl)
                n611 = Multiply(x=w964, y=17179869184.0) -> (x*y=w960:dbl)
                n612 = Multiply(x=50.0, y=w960) -> (x*y=w958:dbl)
                n613 = Divide(x=w958, y=2500000.0) -> (x/y=w961:dbl)
                n614 = Round Toward +Infinity(x=w961) -> (ceil(x): smallest int >= x=w963:dbl)
              }
              frame 7 {
                n615 = local read "H1 Volt"() -> (w974:dbl)
                n616 = local read "H2 order"() -> (w981:dbl)
                n617 = local read "H1 order"() -> (w982:dbl)
                n618 = local read "H2 Volt"() -> (w986:dbl)
                n619 = Power Of X(1:2.0 ("x"), 2:16.0 ("y")) -> (0:w971:dbl)
                n620 = local read "Frequency"() -> (w990:dbl)
                n621 = local read "Voltage"() -> (w991:dbl)
                n622 = local read "H1 Phase"() -> (w989:dbl)
                n623 = local read "H2 Phase"() -> (w993:dbl)
                n624 = Multiply(x=w974, y=52428.8) -> (x*y=w987:dbl)
                n625 = Multiply(x=w986, y=52428.8) -> (x*y=w984:dbl)
                n626 = Round Toward +Infinity(x=w987) -> (ceil(x): smallest int >= x=w973:dbl)
                n627 = Multiply(x=w973, y=360.0) -> (x*y=w970:dbl)
                n628 = Divide(x=w970, y=w971) -> (x/y=w972:dbl)
                n629 = Round Toward +Infinity(x=w984) -> (ceil(x): smallest int >= x=w983:dbl)
                n630 = Format Into String(format string="%02x%02x", w982, w981) -> (resulting string=w979:string)  [unwired: 2 in, 1 out]
                n631 = Hexadecimal String To Number(string=w979) -> (number=w978:u32)  [unwired: 2 in, 1 out]
              }
            }
            n632 = local read "Phase"() -> (w740:dbl)
            n633 = local read "Voltage"() -> (w746:dbl)
            n634 = local read "Phase unit"() -> (w741:u16)
            n635 = case shown="1" w741 {
              tunnel: w740 -> [w838 w843]
              tunnel: [w838 w839] -> w739
              frame 0, Default {
                # "deg"
              }
              frame 1 {
                # "rad->deg"
                n636 = Divide(x=w843, y=6.283185307179586) -> (x/y=w841:dbl)
                n637 = Multiply(x=w841, y=360.0) -> (x*y=w839:dbl)
              }
            }
            n638 = Multiply(x=w804, y=52428.8) -> (x*y=w803:dbl)
            n639 = Power Of X(1:2.0 ("x"), 2:16.0 ("y")) -> (0:w807:dbl)
            n640 = call "Convert dec to hex.vi"("P.u. Voltage"=w829) -> ("Numeric"=w801:dbl)  [unwired: 10 in]
            n641 = Divide(x=w810, y=360.0) -> (x/y=w808:dbl)
            n642 = Round Toward +Infinity(x=w803) -> (ceil(x): smallest int >= x=w742:dbl)
            n643 = Multiply(x=w807, y=w808) -> (x*y=w802:dbl)
            n644 = To Long Integer(number=w802) -> (32bit integer=w797:i32)
            n645 = To Long Integer(number=w801) -> (32bit integer=w799:i32)
            n646 = To Long Integer(number=w742) -> (32bit integer=w798:i32)
            n647 = To Long Integer(number=w778) -> (32bit integer=w777:i32)
            n648 = To Long Integer(number=w776) -> (32bit integer=w775:i32)
            n649 = To Long Integer(number=w774) -> (32bit integer=w773:i32)
            n650 = To Long Integer(number=w772) -> (32bit integer=w771:i32)
            n651 = Format Into String(format string="%1x%1x%6x%4x%4x%4x%04x%04x%04x", "Data type", w779, w799, w798, w797, w777, w775, w773, w771) -> (resulting string=w758:string)  [unwired: 2 in, 1 out]
            "resulting string 2" <- w758
            n652 = String Subset(string=w758, offset (0)=0, length (rest)=4 ("length (rest)")) -> (substring=w753:string)
            n653 = String Subset(string=w758, offset (0)=4, length (rest)=4 ("length (rest)")) -> (substring=w788:string)
            n654 = String Subset(string=w758, offset (0)=8, length (rest)=4 ("length (rest)")) -> (substring=w787:string)
            n655 = String Subset(string=w758, offset (0)=12, length (rest)=4 ("length (rest)")) -> (substring=w766:string)
            n656 = String Subset(string=w758, offset (0)=16, length (rest)=4 ("length (rest)")) -> (substring=w764:string)
            n657 = Bundle(0, 0) -> (w747:cluster{i32, i32})  [unwired: 1 in]
            n658 = String Subset(string=w758, offset (0)=20, length (rest)=4 ("length (rest)")) -> (substring=w762:string)
            n659 = String Subset(string=w758, offset (0)=28, length (rest)=4 ("length (rest)")) -> (substring=w756:string)
            n660 = String Subset(string=w758, offset (0)=24, length (rest)=4 ("length (rest)")) -> (substring=w757:string)
            n661 = Hexadecimal String To Number(string=w753) -> (number=w770:u32)  [unwired: 2 in, 1 out]
            n662 = Hexadecimal String To Number(string=w788) -> (number=w769:u32)  [unwired: 2 in, 1 out]
            n663 = Hexadecimal String To Number(string=w787) -> (number=w786:u32)  [unwired: 2 in, 1 out]
            n664 = Hexadecimal String To Number(string=w766) -> (number=w785:u32)  [unwired: 2 in, 1 out]
            n665 = Hexadecimal String To Number(string=w764) -> (number=w763:u32)  [unwired: 2 in, 1 out]
            n666 = Hexadecimal String To Number(string=w762) -> (number=w761:u32)  [unwired: 2 in, 1 out]
            n667 = Hexadecimal String To Number(string=w757) -> (number=w755:u32)  [unwired: 2 in, 1 out]
            n668 = Hexadecimal String To Number(string=w756) -> (number=w754:u32)  [unwired: 2 in, 1 out]
            n669 = String To IP(1:"LAN Module IP Address") -> (0:w837:u32)
            n670 = Bundle("Voltage"=w746, "Phase"=w739) -> (w820:cluster{"Voltage ":dbl, "Phase ":dbl})  [unwired: 1 in]
            n671 = Compound Arithmetic op=ADD(w770, w769, w786, w785, w763, w761, w755, w754) -> (w782:u32)
            n672 = Build Array(w747, w820) -> (w821:cluster{"Voltage ":dbl, "Phase ":dbl}[])
            n673 = Number To Hexadecimal String(2:w782) -> (0:w781:string)  [unwired: 1 in]
            n674 = UDP Open(11:u16 40000 ("port")) -> (port=w834:refnum<k16>, 0:w833:errorcluster)  [unwired: 4 in, 1 out]
            n675 = String Subset(string=w781, offset (0)=1, length (rest)=4 ("length (rest)")) -> (substring=w780:string)
            n676 = Format Into String(format string="%01x%01x%06x%04x%04x%04x%04x%04x%04x%04s", "Data type", w779, w801, w742, w802, w778, w776, w774, w772, w780) -> (resulting string=w806:string)  [unwired: 2 in, 1 out]
            "Transmitted Data" <- w806
            n677 = String Length(string=w806) -> (length=w824:i32)
            n678 = Scale By Power Of 2(n=-1, x=w824) -> (x*2^n=w822:i32)
            n679 = for {
              N: w822 -> [_]
              shift-right: [w848] -> _
              shift-left: u32 0 -> [w849]
              tunnel: w806 -> [w847]
              tunnel: w827 -> [w846]
              tunnel: [w845] -> w826 mode=indexing
              tunnel: "%02x" ("format string") -> [w844]
              n680 = Scan From String(format string=w844, input string=w847, initial scan location=w849, default 1=w846) -> (offset past scan=w848:u32, output 1=w845:u8)  [unwired: 1 in, 2 out]
            }
            n681 = Type Cast(x=w826) -> (*(type *) &x=w805:string)  [unwired: 1 in]
            n682 = UDP Write(address=w837, port or service name="LAN Port", connection ID=w834, data in=w805, 8:w833) -> (error out=w836:errorcluster, 3:w835:refnum<k16>)  [unwired: 1 in]
            n683 = UDP Close(connection ID=w835, 8:w836) -> ()  [unwired: 2 out]
            n684 = property on="Phase 2" class="Pict"() -> ("Draw Area Size"=w819:T3)  [unwired: 2 in, 2 out]
            n685 = call <vilib>:"Polar Plot with Point Options.vi"("picture"=picture data[5B], "data array [mag, phase (deg)]"=w821, "dimensions (w,h)"=w819, "polar attributes"=T2 {"maximum"=0.0, "minimum"=0.0, "clip to min"=FALSE, "log?(F)"=FALSE, "grid color"=6710886, "plot color"=65280, "fmt and prec"={"format"=enum."Decimal", "precision"=2}, "visible section"=8}, "Lines/Points"=enum16{"Lines", "Points"}."Lines", "Size"=u16 5) -> ("new picture"=→"Phase 2":picture)  [unwired: 9 in]
          }
        }
      }
    }
    n686 = property on="Select test type" class="Ring (strict)"() -> ("RingText.Text"=w71:string)  [unwired: 2 in, 2 out]
    n687 = Wait (ms)(milliseconds to wait=u32 100) -> ()  [unwired: 1 out]
    n688 = TDMS Set Properties(5:w71, 7:"description", 8:w34, 11:w35) -> (0:w46:errorcluster, 3:w45:refnum<k34>)  [unwired: 2 in, 2 out]
    n689 = TDMS Set Properties(5:"s" ("channel name"), 7:"unit_string" ("channel name"), 8:w46, 9:"Time" ("channel name"), 10:w44, 11:w45) -> (0:w50:errorcluster, 3:w54:refnum<k34>)  [unwired: 2 out]
    n690 = local read "Phase unit"() -> (w33:u16)
    n691 = TDMS Set Properties(5:"volt" ("channel name"), 7:"unit_string" ("channel name"), 8:w50, 9:"Voltage" ("channel name"), 10:w44, 11:w54) -> (0:w49:errorcluster, 3:w53:refnum<k34>)  [unwired: 2 out]
    n692 = case shown="0, Default" w33 {
      tunnel: ["deg" ("channel name") "rad" ("channel name")] -> w32
      frame 0, Default {
      }
      frame 1 {
      }
    }
    n693 = TDMS Set Properties(5:w32, 7:"unit_string" ("channel name"), 8:w49, 9:"Phase" ("channel name"), 10:w44, 11:w53) -> (0:w48:errorcluster, 3:w52:refnum<k34>)  [unwired: 2 out]
    n694 = TDMS Set Properties(5:"Hz" ("channel name"), 7:"unit_string" ("channel name"), 8:w48, 9:"Frequency" ("channel name"), 10:w44, 11:w52) -> (0:w47:errorcluster, 3:w51:refnum<k34>)  [unwired: 2 out]
    n695 = TDMS Set Properties(5:"Hz/s" ("channel name"), 7:"unit_string" ("channel name"), 8:w47, 9:"ROCOF" ("channel name"), 10:w44, 11:w51) -> (0:w38:errorcluster, 3:w39:refnum<k34>)  [unwired: 2 out]
    n696 = Stop(stop? (T)="stop") -> ()
    "Numeric" <- w69
  }
  n697 = disable-structure shown="Enabled" {
    frame Disabled {
      n698 = while {
        stop <- w994 stop-if-true
        w994 = FALSE ("stop? (T)")
        n699 = event shown="[0] \"Voltage step\", \"Frequency step\", \"Start\": Value Change" {
          selector: _ -> [_ _]
          dyn-events: _ -> [_ _]
          timeout: _ -> [_ _]
          event "Voltage step", "Frequency step", "Start": Value Change {
            n700 = event-data() -> ()  [unwired: 1 in, 6 out]
            n701 = local write "Data type"(9 ("Data type")) -> ()
          }
          event "Start": Key Repeat {
            n702 = event-data() -> ()  [unwired: 1 in, 1 out]
          }
        }
        n703 = Stop(stop? (T)=w994) -> ()
      }
    }
    frame Enabled {
    }
  }
  n704 = TDMS Close(8:w18, 11:w17) -> (0:w20:errorcluster, 3:w19:path)
  n705 = call <vilib>:"TDMS - File Viewer (NXG Style).vi"("error in"=w20, "file in"=w19) -> ("error out"=w21:errorcluster)  [unwired: 8 in, 1 out]
  n706 = call <vilib>:"Simple Error Handler.vi"("error in (no error)"=w21) -> ()  [unwired: 4 in, 5 out]
